vi "Measurement.vi"(0 "Position":T3(array[cluster]) {"Z" format="%.1f"; "Y" format="%.1f"; "X" format="%.1f"}, 1 "setup":T4=enum."Show Setup", 2 "Post Process":T2, 4 "File":T5, 5 "Results file":path, 7 "Raw data file":path, 11 "Setup filename":string) -> (14 "2nd plot":cluster{"X array":dbl[], "Y array":dbl[]}[](graph), 19 "Status Out":T1)   [LabVIEW 2013]
uses:
  Anemometry Sub Vis/Controls/Save_Data.ctl
  Anemometry Sub Vis/Controls/Setup.ctl
  Anemometry Sub Vis/Controls/Graph_Type.ctl
  Anemometry Sub Vis/Controls/Post_Process.ctl
  Anemometry Sub Vis/Gen Trav/Multi_Run_Status.ctl
  Anemometry Sub Vis/Controls/Inst_type.ctl
  ADAM Client/Sub VIs/ADAM Controls/Traverse_Level_State.ctl
  Anemometry Sub Vis/File/Setup_Filetype.ctl
  Anemometry Sub Vis/Globals/Trav_pos_global.vi
  Anemometry Sub Vis/Globals/Meas_global.vi
  Anemometry Sub Vis/Acquisition/PWA/PWAtasksGLOBAL.vi
  Anemometry Sub Vis/Acquisition/Data_Translation/DataTranslation_global.vi
  Anemometry Sub Vis/Globals/Preference_global.vi
  Anemometry Sub Vis/Globals/LDA_meas_global_1.vi
  Anemometry Sub Vis/Globals/LDA_meas_global_2.vi
  Anemometry Sub Vis/Globals/Dynamic_call_global.ph.vi
  Anemometry Sub Vis/Globals/Plug_in_data_global.vi
  Anemometry Sub Vis/Globals/Constants_global.vi
panel:
  out "Pause message":string
  out "Statistics":string[][](table)
  out "Actual Sampling freq":dbl=100.0 format="%.1f"
  in  "Desired Sampling freq (Hz)":dbl=100.0 format="%.1f"
  out "Current Block No":i32=5 caption="Current Block"
  in  "Pause":bool
  in  "No of Blocks":i32=5
  in  "stop":bool
  in  "No of samples":i32=1000 min=0 step=1
  in  "PP next block":bool
  in  "Tab Control":T6(tab)
  in  "Second Graph":T8={"Plot 1"=2, "Plot 2"=1, "Save graph"=0, "Plot Type"=enum."Vel histogram"} {"Save graph" items=["Do not save plot", "Save plot"]; "Plot 2" items=["Nothing", "U", "Volts", "Voltsr"]; "Plot 1" items=["Nothing", "U", "Volts", "Voltsr"]}
  in  "First Graph":T8={"Plot 1"=1, "Plot 2"=2, "Save graph"=0, "Plot Type"=enum."Velocity trace"} {"Save graph" items=["Do not save plot", "Save plot"]; "Plot 2" items=["Nothing", "U", "Volts", "Voltsr"]; "Plot 1" items=["Nothing", "U", "Volts", "Voltsr"]}
  out "First plot":cluster{"X array":dbl[], "Y array":dbl[]}[](graph)
  in  "Comments":string
  out "uv":dbl[][](graph)=[[-0.041806189081711534, -0.046435429052714985, -0.04035660097427599, -0.042187605126076694, -0.042052555599004206]]
  out "u^4":dbl[][](graph)
  out "u^3":dbl[][](graph)
  out "u^2":dbl[][](graph)=[[0.09743628875280319, 0.10575821456272283, 0.10126262927293661, 0.09890442087602569, 0.1022948212436432]]
  out "U":dbl[][](graph)=[[0.8295029456391334, 0.8915896983798417, 0.8415763502225625, 0.8394746126219594, 0.8466062785395404]]
  in  "Block average display control":cluster{"Name":string, "Include":bool}[](array[cluster])=[{"Name"="FF (C)", "Include"=FALSE}]
  in  "No of bins in histogram":i32=100
  out "Measurement time (min)":dbl=6.0 format="%.2f"
  in  "Correlate?":T9(ring)
  out "Diagnostic info":string[][](table)
  out "Array U":dbl[][](array[numeric]) format="%.2e"
  out "Array u^2":dbl[][](array[numeric]) format="%.2e"
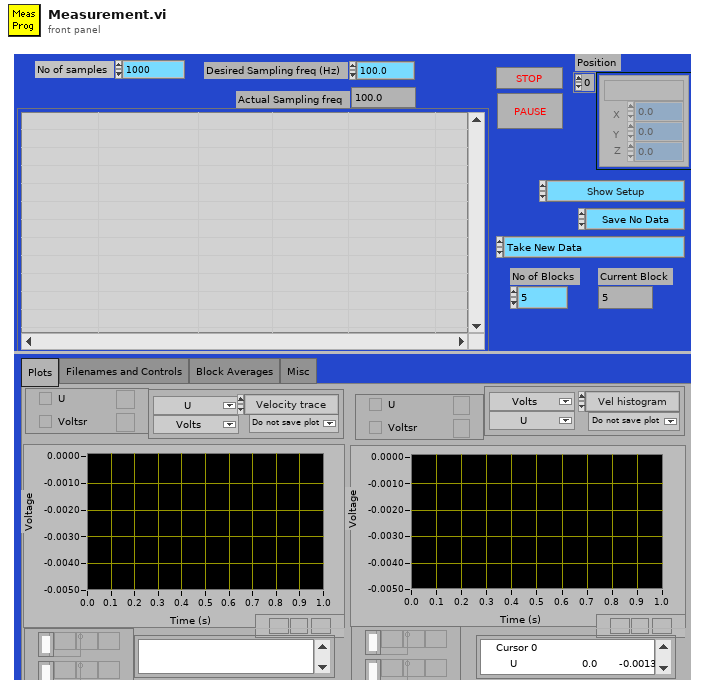
[diagram p1: front panel]
types:
  T1 = typedef "Multi_Run_Status.ctl" = enum16{"Continue", "Jump to Next Point", "Jump to Next Row", "Jump To Fall Back", "Terminate Run"}
  T2 = typedef "Post_Process.ctl" = enum16{"Take New Data", "Post Process Raw Data File"}
  T3 = cluster{"Name":string, "X":dbl, "Y":dbl, "Z":dbl}[]
  T4 = typedef "Setup.ctl" = enum16{"Run Program", "Show Setup", "Save Current Setup", "Setup Front Panel"}
  T5 = typedef "Save_Data.ctl" = enum16{"Save No Data", "Save Data"}
  T6 = enum32{"Plots", "Filenames and Controls", "Block Averages", "Misc"}
  T7 = typedef "Graph_Type.ctl" = enum16{"Show no graph", "Voltage trace", "Velocity trace", "Vel histogram", "Spectrum", "f.E(f) v Log f", "Auto-Corr"}
  T8 = cluster{"Plot 1":u16, "Plot 2":u16, "Save graph":u16, "Plot Type":T7}
  T9 = enum16{"Cross correlation off", "Show correlation panel", "Correlate without activating panel"}
  T10 = enum32{"Bad", "Idle", "Run top level", "Running"}
  T11 = cluster{"Name":string, "X":dbl, "Y":dbl, "Z":dbl}
  T12 = enum16{"Velocity", "Transit time", "Arrival time"}
  T13 = enum16{"Save no data", "Save data in new files", "Save data in existing files"}
  T14 = enum16{"Zero or one", "One", "Zero or more", "One or more"}
  T15 = cluster{"Weighting":dbl[], "Time (ms)":dbl[], "Voltage":dbl[], "Eng Values":dbl[]}
  T16 = typedef "Inst_type.ctl" = enum16{"Propeller anemometer", "Raw voltage", "Pressure Transducer", "Pitot-static tube", "Preston tube", "Hot wire", "Cross wire 1", "Cross wire 2", "Generic Linear", "Generic Polynomial", "Generic BackPoly", "Fast FID", "Thermocouple", "Cold wire", "Pulsed Wire", "LDA Vel", "LDA Tran time", "LDA Arr time"}
  T17 = typedef "Traverse_Level_State.ctl" = enum16{"Running", "Complete"}
  T18 = typedef "Setup_Filetype.ctl" = enum16{"Measurement Setups", "Calibration Setups", "General", "Results File Plotter Setups", "Speed Calib Tweaks"}
  T19 = typedef "Traverse_cluster.ctl" = cluster{"Start X":dbl, "Start Y":dbl, "Start Z":dbl, "End X":dbl, "End Y":dbl, "End Z":dbl, "No. of pts.":i32, "Spacing":T20, "Filename":path, "Tunnel Speed":dbl, "Averaging time (min)":dbl, "Extra Commands":string, "Specific Arguments":string, "Emission Rate (l/min)":dbl, "Trace Gas Concentration (%)":dbl, "Density Ratio":string, "Comments":string, "Row No":i32, "Row Type Selector":T21, "Completion time":string, "Row Duration (mins)":dbl, "No. of Valid pts.":i32, "Meas Setup File":string}
  T20 = typedef "Spacing.ctl" = enum16{"Linear", "Log", "Gauss", "Specified", "N/A"}
  T21 = typedef "Multi_run_mode.ctl" = enum16{"Move Traverse Only", "Set Tunnel Speed Only", "Set Source Only", "Set Measurement Conditions", "Single Measurement", "Vertical Profile", "Lateral Profile", "Longitudinal Profile", "Explore Volume", "Multi-Axis Profile", "Auto Calibrate", "Meas Fast FID Bkgnd", "Check Beam Power", "Scanning Valve Measurement", "Run VI Named:", "Set ADAM Ch", "Wait (minutes)", "Send Message", "Synchronize With:", "Fall Back to this Row", "Turn Off Row Repeating", "Blank Row", "Traverse 3D Volume"}
  T22 = typedef "Analysis_info_cluster.ctl" = cluster{"Colour":u32, "Inst type":T16, "Inst name":string, "Symbol":string, "Code name":string, "Extra Info":string, "Inst Array":T23, "Extra Titles":string[], "Extra Values":string[], "U":dbl, "u^2":dbl, "u^3":dbl, "u^4":dbl, "Skew_u":dbl, "Kurt_u":dbl, "Sd Error in Mean":dbl, "% u'/U":dbl, "X":dbl, "Y":dbl, "Z":dbl, "Timescale integral to 25%":dbl, "Sd Error in Variance":dbl, "Calib File":path, "Calib Constants":dbl[], "Output Position":bool, "Full Stats":bool, "Av Sampling Rate":dbl, "Av No of Samples":dbl, "Total Meas Time (s)":dbl, "ADAM Ch Name":string}
  T23 = typedef "Instrument_Array.ctl" = enum16{"PWA", "LDA", "Analogue"}
  T24 = typedef "LDA_Setup.ctl" = cluster{"dimensions":enum16{"1D", "2D"}, "Analogue Freq Multiplier":dbl}
  T25 = enum16{"Velocity", "Transit time", "Arrival time"}[]
  T26 = typedef "BSA_Type.ctl" = enum16{"57N11", "BSA F60"}
  T27 = typedef "BSA_info_Cluster.ctl" = cluster{"GPIB Address":string, "No of Check Bytes":i32, "Extra Info":string, "COLOUR":u32, "Wavelength (nm)":dbl}
  T28 = typedef "Ch_and_Spans.ctl" = cluster{"high limit (10V)":sgl, "low limit (-10V)":sgl, "Ch No":i16, "Var name":string, "Use Latest Calib":bool, "DAQmx Chan":tag}
  T29 = cluster{"Weighting":dbl[], "Time (ms)":dbl[], "Voltage":dbl[], "Eng Values":dbl[]}[]
  T30 = cluster{"Insts for plotting[0]":u16, "Insts for plotting[1]":u16}
  T31 = typedef "PWA_Data.ctl" = enum16{"No PWA Data", "One Ch PWA"}
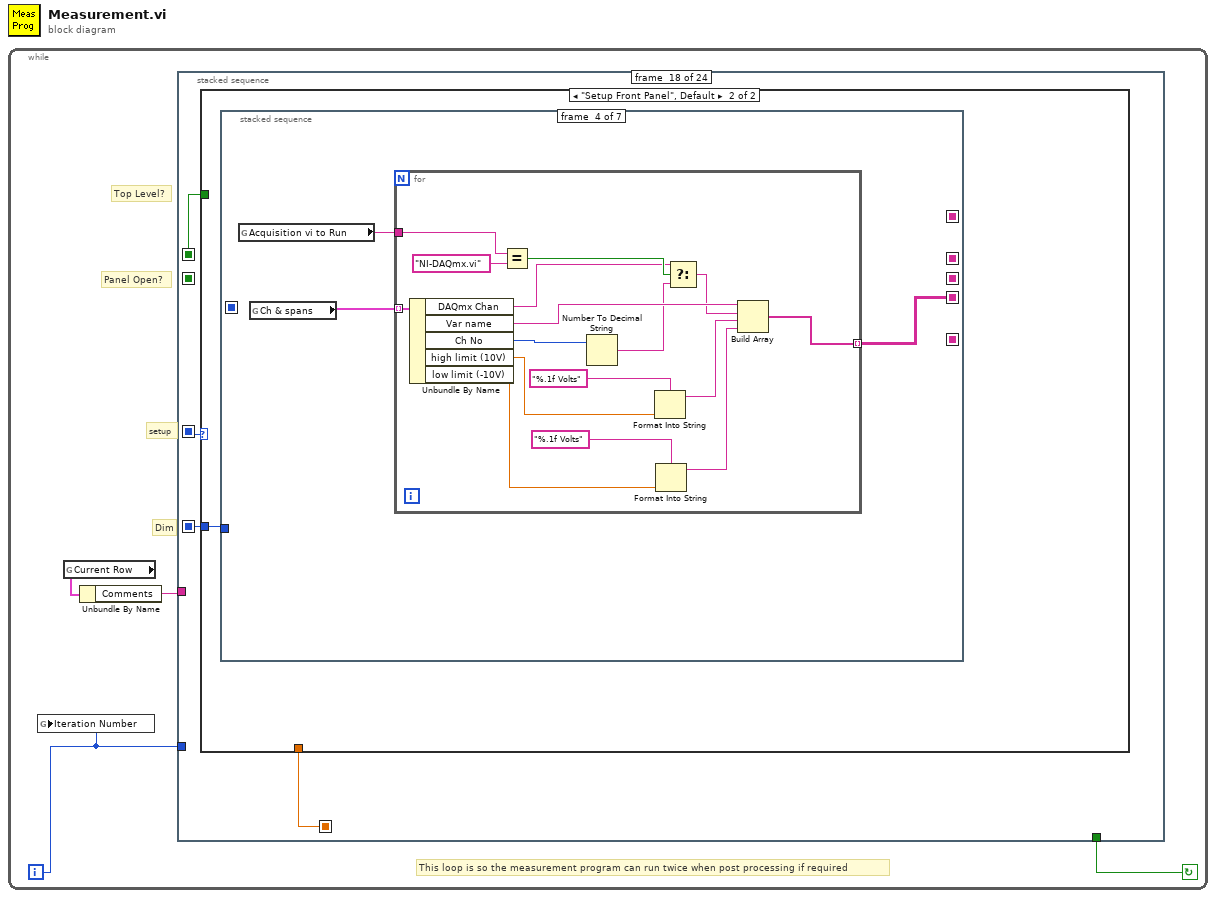
[diagram p0: block diagram]
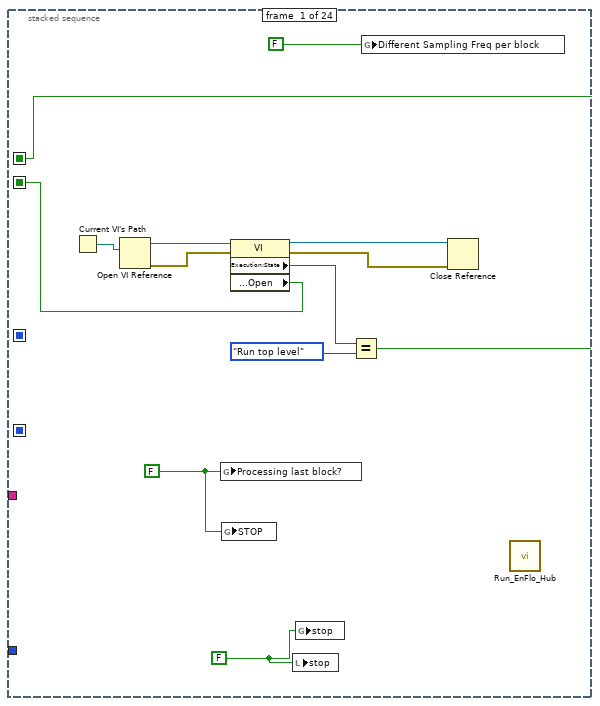
[diagram p2: hidden frame]
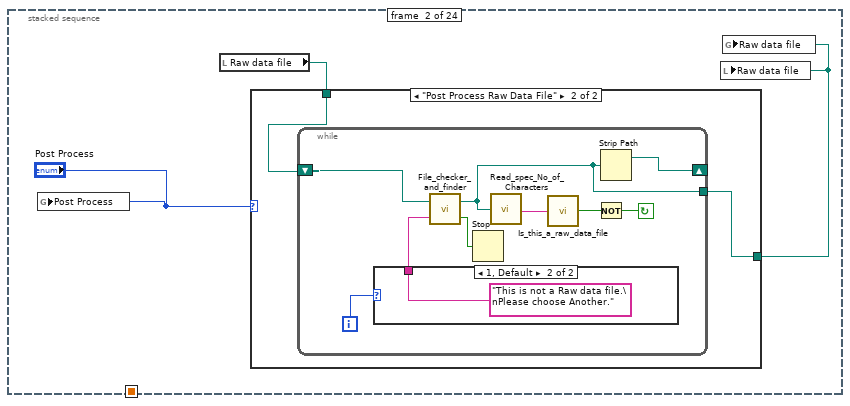
[diagram p3: hidden frame]
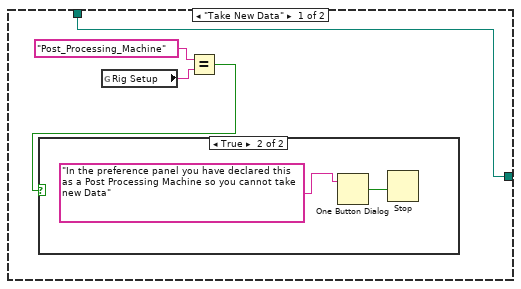
[diagram p4: hidden frame]
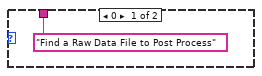
[diagram p6: hidden frame]
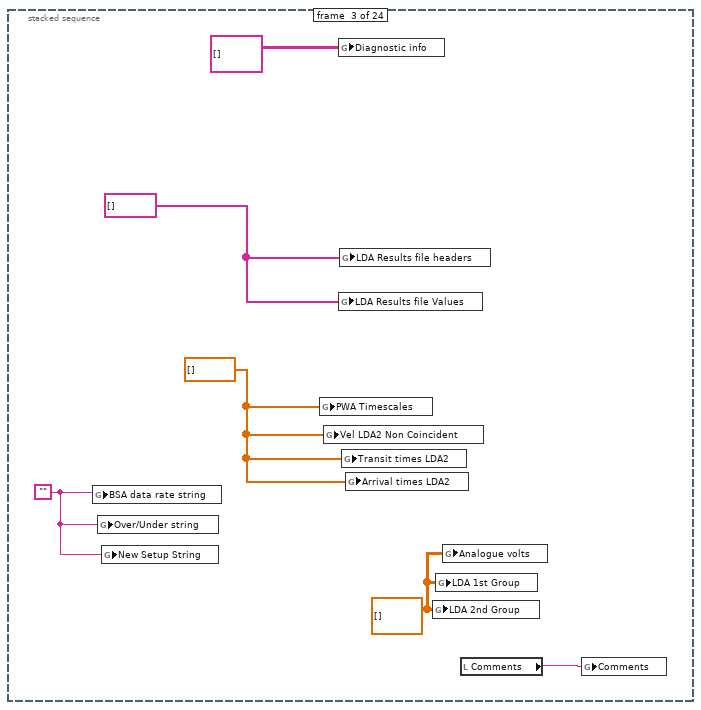
[diagram p7: hidden frame]
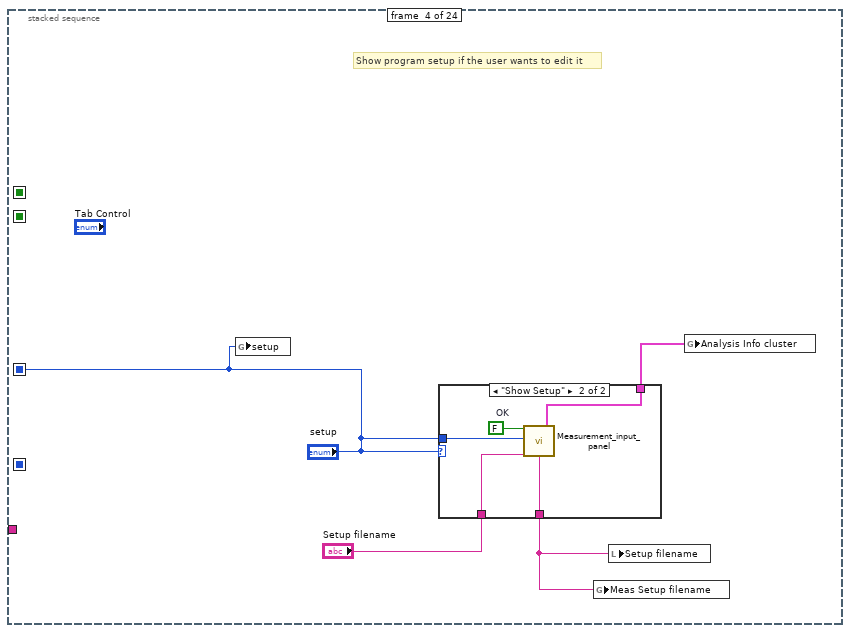
[diagram p8: hidden frame]
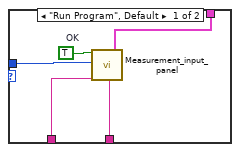
[diagram p9: hidden frame]
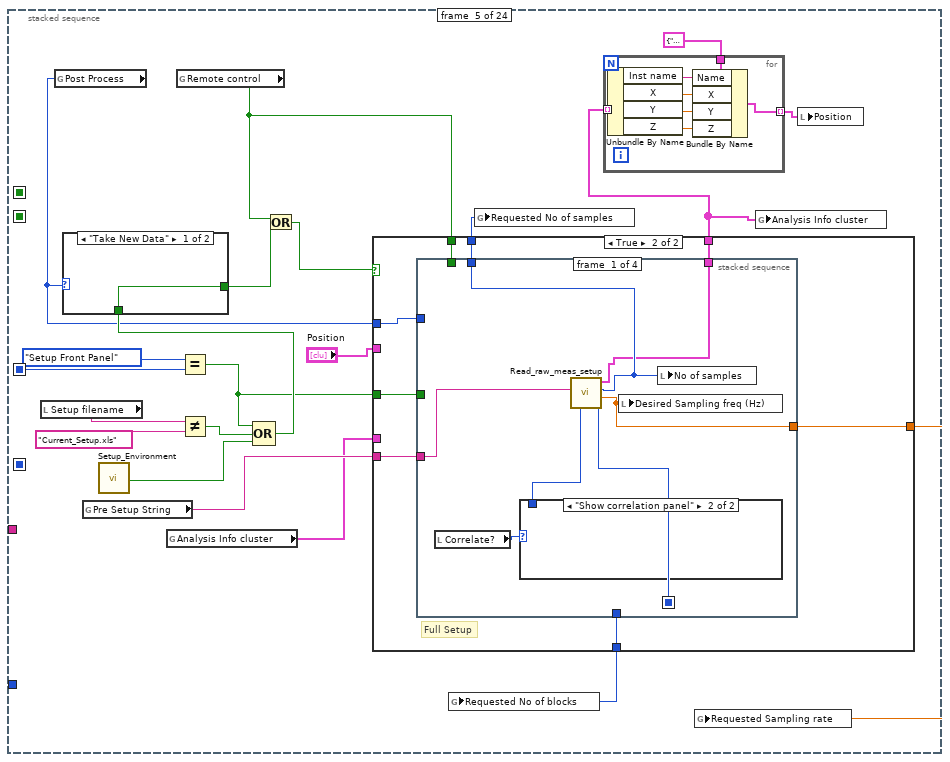
[diagram p10: hidden frame]
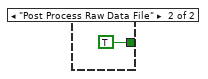
[diagram p11: hidden frame]
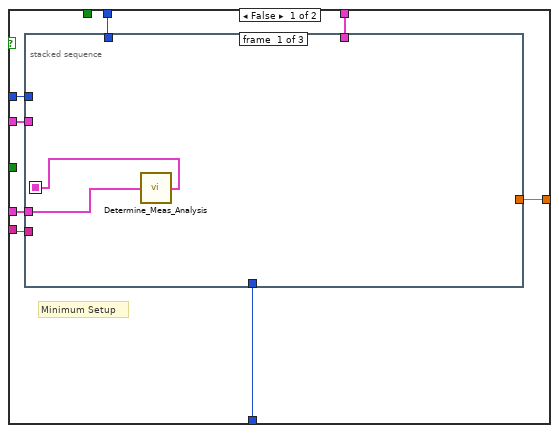
[diagram p12: hidden frame]
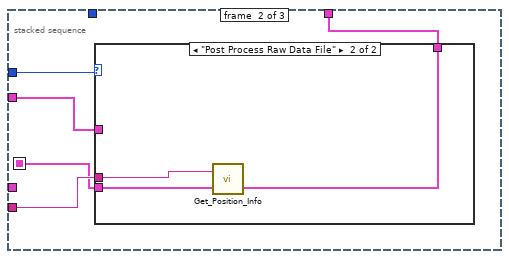
[diagram p13: hidden frame]
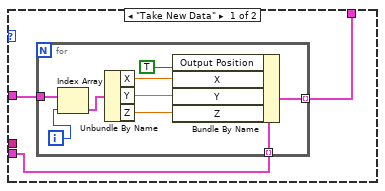
[diagram p14: hidden frame]
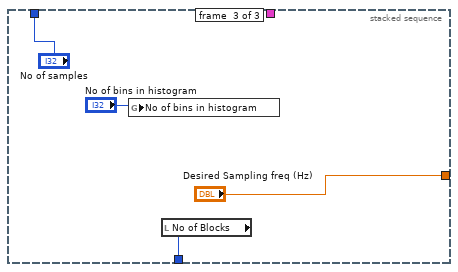
[diagram p15: hidden frame]
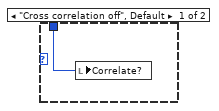
[diagram p16: hidden frame]
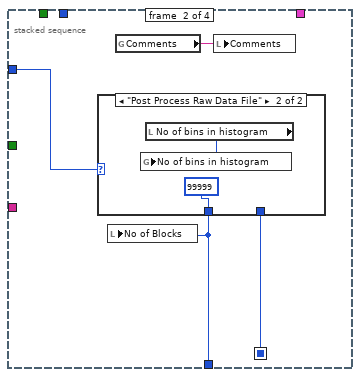
[diagram p17: hidden frame]
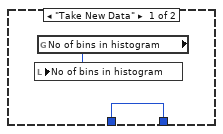
[diagram p18: hidden frame]
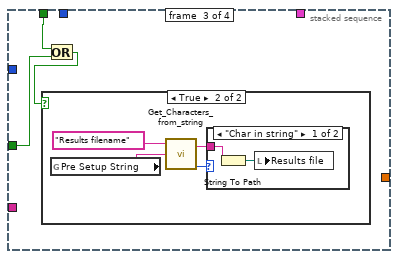
[diagram p19: hidden frame]
diagram:
  n1 = while {
    i -> [w1]
    stop <- w2 continue-if-true
    # "This loop is so the measurement program can run twice when post processing if required"
    # "Panel Open?"
    # "Top Level?"
    # "setup"
    # "Dim"
    n2 = global write "Meas_global.vi" "Iteration Number"(w1) -> ()
    n3 = global read "Trav_pos_global.vi" "Current Row"() -> (w3:T19)
    n4 = Unbundle By Name(w3) -> ("Comments"=w4:string)
    n5 = stacked-sequence {
      seq-local: [_ _ _ _ _ _ _ _ w202 _ _ _ _ _ _ _ _ _ _ _ _ _ _ _] -> [_ _ _ _ _ _ _ _ _ _ _ _ _ _ _ _ _ w752 _ _ _ _ _ _]
      seq-local: [_ _ _ "setup" _ _ _ _ _ _ _ _ _ _ _ _ _ _ _ _ _ _ _ _] -> [_ _ _ _ w71 _ _ _ w200 w289 _ _ _ _ w662 w682 w689 w753 w960 w1010 w1065 _ _ w1171]
      seq-local: [_ _ _ _ _ _ _ _ _ _ _ _ _ _ _ _ w685 _ _ _ _ _ _ _] -> [_ _ _ _ _ _ _ _ _ _ _ _ _ _ _ _ _ w751 w950 _ _ _ _ _]
      seq-local: [w7 _ _ _ _ _ _ _ _ _ _ _ _ _ _ _ _ _ _ _ _ _ _ _] -> [_ _ _ _ _ _ _ _ _ w269 _ _ _ _ w658 _ _ w750 _ _ _ _ _ _]
      seq-local: [w6 _ _ _ _ _ _ _ _ _ _ _ _ _ _ _ _ _ _ _ _ _ _ _] -> [_ _ _ _ _ _ _ _ _ _ _ _ w481 _ _ _ _ _ _ _ _ _ _ _]
      tunnel: w4 -> [_ _ _ _ _ _ _ w197 _ _ _ _ _ _ _ _ _ _ _ _ _ _ w1140 _]
      tunnel: w1 -> [_ _ _ _ _ _ _ _ _ _ _ _ _ _ _ _ _ _ _ _ _ _ w1135 _]
      tunnel: [_ _ _ _ _ _ _ _ _ _ _ _ _ _ _ _ _ _ _ _ _ _ w1134 _] -> w2
      frame #0 {
        w15 = FALSE ("Processing last block?")
        w16 = FALSE ("stop")
        n6 = Current VI's Path() -> (path=w8:path)
        n7 = Open VI Reference(vi path=w8) -> (vi reference=w9:refnum<vi>, error out=w10:errorcluster)  [unwired: 1 in, 4 out]
        n8 = global write "Meas_global.vi" "Processing last block?"(w15) -> ()
        n9 = global write "PWAtasksGLOBAL.vi" "STOP"(w15) -> ()
        n10 = property class="VI"(reference=w9, error in=w10) -> (reference out=w11:refnum<vi>, error out=w12:errorcluster, "Execution:State"=w13:T10, "Front Panel.Open"=w6:bool)
        n11 = local write "stop"(w16) -> ()
        n12 = global write "Meas_global.vi" "stop"(w16) -> ()
        n13 = Equal?(x=w13, y=T10."Run top level" ("Exec.State")) -> (x = y?=w7:bool)
        n14 = global write "DataTranslation_global.vi" "Different Sampling Freq per block"(FALSE ("Different Sampling Freq per block")) -> ()
        n15 = Close Reference(reference=w11, error in (no error)=w12) -> ()  [unwired: 1 out]
        n16 = call "Run_EnFlo_Hub.vi"() -> ()  [unwired: 8 out]
      }
      frame #1 {
        n17 = global write "Meas_global.vi" "Post Process"("Post Process") -> ()
        n18 = local read "Raw data file"() -> (w19:path)
        n19 = case shown="\"Post Process Raw Data File\"" "Post Process" {
          tunnel: [w23 w27] -> w18
          tunnel: w19 -> [w23 w26]
          frame "Take New Data" {
            n20 = global read "Preference_global.vi" "Rig Setup"() -> (w22:string)
            n21 = Equal?(x="Post_Processing_Machine" ("Rig Setup"), y=w22) -> (x = y?=w20:bool)
            n22 = case shown="True" w20 {
              frame False {
              }
              frame True {
                n23 = One Button Dialog(message="In the preference panel you have declared this as a Post Processing Machine so you cannot take new Data") -> (true=w24:bool)  [unwired: 1 in]
                n24 = Stop(stop? (T)=w24) -> ()
              }
            }
          }
          frame "Post Process Raw Data File" {
            n25 = while {
              tunnel: [w29] -> w27
              shift-left: w26 -> [w31]
              shift-right: [w30] -> _
              i -> [w32]
              stop <- w33 continue-if-true
              n26 = case shown="1, Default" w32 {
                tunnel: ["Find a Raw Data File to Post Process" ("Promp if not found") "This is not a Raw data file.\nPlease choose Another." ("Promp if not found")] -> w36
                frame 0 {
                }
                frame 1, Default {
                }
              }
              n27 = call "File_checker_and_finder.vi"("Promp if not found"=w36, "Filename In"=w31) -> ("cancelled"=w28:bool, "Filename Out"=w29:path)
              n28 = Stop(stop? (T)=w28) -> ()
              n29 = call "Read_spec_No_of_Characters.vi"("Filename"=w29) -> ("character string"=w35:string)  [unwired: 1 out]
              n30 = call "Is_this_a_raw_data_file.vi"("character string"=w35) -> ("Raw Dat File?"=w34:bool)  [unwired: 2 out]
              n31 = Not(x=w34) -> (.not. x?=w33:bool)
              n32 = Strip Path(path=w29) -> (stripped path=w30:path)  [unwired: 1 out]
            }
          }
        }
        n33 = local write "Raw data file"(w18) -> ()
        n34 = global write "Meas_global.vi" "Raw data file"(w18) -> ()
      }
      frame #2 {
        w39 = dbl[][] [] ("LDA 2nd Group")
        w40 = dbl[] [] ("LDA Timescales")
        w42 = string[] [] ("Plug in values")
        w44 = ""
        n35 = global write "Meas_global.vi" "BSA data rate string"(w44) -> ()
        n36 = global write "Meas_global.vi" "Over/Under string"(w44) -> ()
        n37 = global write "Meas_global.vi" "New Setup String"(w44) -> ()
        n38 = global write "PWAtasksGLOBAL.vi" "PWA Timescales"(w40) -> ()
        n39 = global write "LDA_meas_global_2.vi" "Vel LDA2 Non Coincident"(w40) -> ()
        n40 = global write "Meas_global.vi" "Diagnostic info"(string[][] [] ("Diagnostic info")) -> ()
        n41 = global write "LDA_meas_global_1.vi" "LDA Results file Values"(w42) -> ()
        n42 = global write "LDA_meas_global_1.vi" "LDA Results file headers"(w42) -> ()
        n43 = global write "LDA_meas_global_2.vi" "Transit times LDA2"(w40) -> ()
        n44 = global write "LDA_meas_global_2.vi" "Arrival times LDA2"(w40) -> ()
        n45 = global write "LDA_meas_global_2.vi" "LDA 2nd Group"(w39) -> ()
        n46 = global write "LDA_meas_global_2.vi" "LDA 1st Group"(w39) -> ()
        n47 = global write "Meas_global.vi" "Analogue volts"(w39) -> ()
        n48 = local read "Comments"() -> (w43:string)
        n49 = global write "Meas_global.vi" "Comments"(w43) -> ()
      }
      frame #3 {
        # "Show program setup if the user wants to edit it"
        n50 = global write "Meas_global.vi" "setup"("setup") -> ()
        n51 = case shown="\"Show Setup\"" "setup" {
          tunnel: [w52 w57] -> w48
          tunnel: "Setup filename" -> [w51 w56]
          tunnel: [w50 w55] -> w46
          tunnel: "setup" -> [w49 w54]
          frame "Run Program", Default {
            w53 = TRUE  # OK
            n52 = call "Measurement_input_panel.vi"("OK"=w53, "setup"=w49, "Setup filename"=w51) -> ("Setup filename out"=w50:string, "Analysis Info cluster"=w52:T22[])  [unwired: 15 out]
          }
          frame "Show Setup" {
            w58 = FALSE  # OK
            n53 = call "Measurement_input_panel.vi"("OK"=w58, "setup"=w54, "Setup filename"=w56) -> ("Setup filename out"=w55:string, "Analysis Info cluster"=w57:T22[])  [unwired: 15 out]
          }
        }
        n54 = global write "Meas_global.vi" "Meas Setup filename"(w46) -> ()
        n55 = local write "Setup filename"(w46) -> ()
        n56 = global write "Meas_global.vi" "Analysis Info cluster"(w48) -> ()
      }
      frame #4 {
        n57 = local read "Setup filename"() -> (w75:string)
        n58 = global read "Meas_global.vi" "Post Process"() -> (w70:T2)
        n59 = global read "Meas_global.vi" "Pre Setup String"() -> (w66:string)
        n60 = call "Setup_Environment.vi"() -> ("First Time"=w67:bool)  [unwired: 1 in]
        n61 = global read "Meas_global.vi" "Analysis Info cluster"() -> (w63:T22[])
        n62 = global read "Meas_global.vi" "Remote control"() -> (w65:bool)
        n63 = Equal?(x=Setup."Setup Front Panel" ("setup"), y=w71) -> (x = y?=w64:bool)
        n64 = Not Equal?(x=w75, y="Current_Setup.xls" ("Setup filename")) -> (x != y?=w73:bool)
        n65 = Compound Arithmetic op=OR(w64, w73, w67) -> (w72:bool)
        n66 = case shown="\"Take New Data\"" w70 {
          tunnel: [w87 TRUE] -> w79
          tunnel: w72 -> [w87 _]
          frame "Take New Data" {
          }
          frame "Post Process Raw Data File" {
          }
        }
        n67 = Or(x=w65, y=w79) -> (x .or. y?=w78:bool)
        n68 = case shown="True" w78 {
          tunnel: w70 -> [w92 w130]
          tunnel: [w96 w129] -> w68
          tunnel: [w95 w124] -> w77
          tunnel: [w94 w128] -> w76
          tunnel: [w93 w127] -> w62
          tunnel: w66 -> [w91 w126]
          tunnel: "Position" -> [w90 _]
          tunnel: w65 -> [_ w125]
          tunnel: w64 -> [_ w123]
          tunnel: w63 -> [w89 _]
          frame False {
            # "Minimum Setup"
            n69 = stacked-sequence {
              seq-local: [w97 _ _] -> [_ w99 _]
              tunnel: [_ _ "Desired Sampling freq (Hz)"] -> w96
              tunnel: [_ _ w121] -> w95
              tunnel: [_ _ "No of samples"] -> w94
              tunnel: [_ w102 _] -> w93
              tunnel: w92 -> [_ w103 _]
              tunnel: w91 -> [_ w101 _]
              tunnel: w90 -> [_ w100 _]
              tunnel: w89 -> [w98 _ _]
              frame #0 {
                n70 = call "Determine_Meas_Analysis.vi"("Analysis info Cluster In"=w98) -> ("Analysis info Cluster Out"=w97:T22[])
              }
              frame #1 {
                n71 = case shown="\"Post Process Raw Data File\"" w103 {
                  tunnel: [w104 w116] -> w102
                  tunnel: w100 -> [w106 _]
                  tunnel: w101 -> [_ w117]
                  tunnel: w99 -> [w105 w118]
                  frame "Take New Data" {
                    n72 = for {
                      tunnel: w106 -> [w109]
                      tunnel: w105 -> [w115] mode=indexing
                      tunnel: [w111] -> w104 mode=indexing
                      i -> [w110]
                      n73 = Index Array(array=w109, index=w110) -> (element=w108:T11)
                      n74 = Unbundle By Name(w108) -> ("X"=w112:dbl, "Y"=w113:dbl, "Z"=w114:dbl)
                      n75 = Bundle By Name(cluster=w115, "Output Position"=TRUE, "X"=w112, "Y"=w113, "Z"=w114) -> (w111:T22)
                    }
                  }
                  frame "Post Process Raw Data File" {
                    n76 = call "Get_Position_Info.vi"("Analysis Info cluster"=w118, "Setup file string"=w117) -> ("Analysis Info cluster 2"=w116:T22[])  [unwired: 1 in]
                  }
                }
              }
              frame #2 {
                n77 = global write "Meas_global.vi" "No of bins in histogram"("No of bins in histogram") -> ()
                n78 = local read "No of Blocks"() -> (w121:i32)
              }
            }
          }
          frame True {
            # "Full Setup"
            n79 = stacked-sequence {
              seq-local: [w134 _ _ _] -> [_ w140 _ _]
              tunnel: w130 -> [_ w141 _ w156]
              tunnel: [w137 _ _ _] -> w129
              tunnel: [w136 _ _ _] -> w128
              tunnel: [w133 _ _ _] -> w127
              tunnel: w126 -> [w135 _ _ _]
              tunnel: w125 -> [_ _ w149 _]
              tunnel: [_ w139 _ _] -> w124
              tunnel: w123 -> [_ _ w148 _]
              frame #0 {
                n80 = local read "Correlate?"() -> (w132:T9)
                n81 = call "Read_raw_meas_setup.vi"("Setup file string"=w135) -> ("No of Blocks"=w134:i32, "Sampling freq (Hz)"=w137:dbl, "No of samples"=w136:i32, "Analysis Info cluster 2"=w133:T22[], "Correlate?"=w131:T9)  [unwired: 4 out]
                n82 = case shown="\"Show correlation panel\"" w132 {
                  tunnel: w131 -> [w138 _]
                  frame "Cross correlation off", Default {
                    n83 = local write "Correlate?"(w138) -> ()
                  }
                  frame "Show correlation panel" {
                  }
                }
                n84 = local write "Desired Sampling freq (Hz)"(w137) -> ()
                n85 = local write "No of samples"(w136) -> ()
              }
              frame #1 {
                n86 = case shown="\"Post Process Raw Data File\"" w141 {
                  tunnel: [w144 99999 ("No of Blocks")] -> w139
                  tunnel: w140 -> [w144 _]
                  frame "Take New Data" {
                    n87 = global read "Meas_global.vi" "No of bins in histogram"() -> (w143:i32)
                    n88 = local write "No of bins in histogram"(w143) -> ()
                  }
                  frame "Post Process Raw Data File" {
                    n89 = local read "No of bins in histogram"() -> (w145:i32)
                    n90 = global write "Meas_global.vi" "No of bins in histogram"(w145) -> ()
                  }
                }
                n91 = local write "No of Blocks"(w139) -> ()
                n92 = global read "Meas_global.vi" "Comments"() -> (w142:string)
                n93 = local write "Comments"(w142) -> ()
              }
              frame #2 {
                n94 = Or(x=w149, y=w148) -> (x .or. y?=w147:bool)
                n95 = case shown="True" w147 {
                  frame False {
                  }
                  frame True {
                    n96 = global read "Meas_global.vi" "Pre Setup String"() -> (w150:string)
                    n97 = call "Get_Characters_from_string.vi"("Input string"=w150, "Variable name"="Results filename") -> ("Status"=w153:enum16{"Char in string", "Char not in string"}, "Value"=w152:string)  [unwired: 1 in]
                    n98 = case shown="\"Char in string\"" w153 {
                      tunnel: w152 -> [w155 _]
                      frame "Char in string" {
                        n99 = String To Path(string=w155) -> (path=w154:path)
                        n100 = local write "Results file"(w154) -> ()
                      }
                      frame "Char not in string" {
                      }
                    }
                  }
                }
              }
              frame #3 {
                n101 = case shown="\"Take New Data\"" w156 {
                  frame "Take New Data" {
                    n102 = global read "Meas_global.vi" "Second Graph"() -> (w157:T8)
                    n103 = global read "Meas_global.vi" "First Graph"() -> (w158:T8)
                    n104 = local write "Second Graph"(w157) -> ()
                    n105 = local write "First Graph"(w158) -> ()
                  }
                  frame "Post Process Raw Data File" {
                  }
                }
              }
            }
          }
        }
        n106 = global write "Meas_global.vi" "Requested No of blocks"(w77) -> ()
        n107 = global write "Meas_global.vi" "Requested No of samples"(w76) -> ()
        n108 = for {
          tunnel: w62 -> [w86] mode=indexing
          tunnel: [w82] -> w60 mode=indexing
          tunnel: T11 {"Name"="", "X"=0.0, "Y"=0.0, "Z"=0.0} ("Position") -> [w81]
          n109 = Unbundle By Name(w86) -> ("Inst name"=w80:string, "X"=w83:dbl, "Y"=w84:dbl, "Z"=w85:dbl)
          n110 = Bundle By Name(cluster=w81, "Name"=w80, "X"=w83, "Y"=w84, "Z"=w85) -> (w82:T11)
        }
        n111 = global write "Meas_global.vi" "Requested Sampling rate"(w68) -> ()
        n112 = global write "Meas_global.vi" "Analysis Info cluster"(w62) -> ()
        n113 = local write "Position"(w60) -> ()
      }
      frame #5 {
        n114 = global read "Meas_global.vi" "Post Process"() -> (w159:T2)
        n115 = case shown="\"Post Process Raw Data File\"" w159 {
          tunnel: [w162 w163] -> w160
          frame "Take New Data" {
            n116 = Get Date/Time In Seconds() -> (seconds since 1Jan1904=w161:timestamp)
            n117 = To Double Precision Float(number=w161) -> (double precision float=w162:dbl)
          }
          frame "Post Process Raw Data File" {
            n118 = global read "Meas_global.vi" "Pre Setup String"() -> (w166:string)
            n119 = call "Get_Characters_from_string.vi"("Input string"=w166, "Variable name"="Seconds since 1/1/04") -> ("Value"=w164:string)  [unwired: 1 in, 1 out]
            n120 = call "String_2_Number.vi"("Value"=w164) -> ("Numeric"=w163:dbl)
          }
        }
        n121 = global write "Meas_global.vi" "Time Data was Aquired"(w160) -> ()
      }
      frame #6 {
        n122 = global read "Dynamic_call_global.ph.vi" "Initial Plug Ins"() -> (w168:string[])
        n123 = global read "Dynamic_call_global.ph.vi" "Initial Plug Ins Extra"() -> (w169:string[])
        n124 = Build Array (concatenate)(w169, w168) -> (w167:string[])
        n125 = Array Size(array=w167) -> (size(s)=w171:i32)
        n126 = Greater Than 0?(x=w171) -> (x > 0?=w170:bool)
        n127 = case shown="True" w170 {
          tunnel: w167 -> [_ w172]
          frame False {
          }
          frame True {
            n128 = stacked-sequence {
              tunnel: w172 -> [w174 _]
              frame #0 {
                n129 = global read "Meas_global.vi" "Post Process"() -> (w176:T2)
                n130 = call "Plug_in_Directories.vi"() -> ("Initial"=w173:path)  [unwired: 3 out]
                n131 = Equal?(x=w176, y=Post_Process."Post Process Raw Data File" ("Post Process")) -> (x = y?=w175:bool)
                n132 = for {
                  tunnel: w175 -> [w182]
                  tunnel: w174 -> [w179] mode=indexing
                  tunnel: w173 -> [w178]
                  w189 = FALSE  # Dialog Box (T)
                  n133 = Build Path(base path=w178, name or relative path=w179) -> (appended path=w180:path)
                  n134 = Open VI Reference(vi path=w180) -> (vi reference=w187:refnum<vi>, error out=w186:errorcluster)  [unwired: 2 in, 3 out]
                  n135 = property class="VI"(reference=w187, error in=w186, "Front Panel Window:Open"=TRUE ("Wait until done")) -> (reference out=w185:refnum<vi>, error out=w184:errorcluster)
                  n136 = invoke class="VI" method="Run VI"(reference=w185, error in=w184, "Wait until done"=w182, "Auto Dispose Ref"=FALSE) -> (reference out=w192:refnum<vi>, error out=w191:errorcluster)  [unwired: 1 in, 3 out]
                  n137 = Close Reference(reference=w192, error in (no error)=w191) -> (error out=w190:errorcluster)
                  n138 = call "EnFlo_Error_Handler.vi"("error in (no error)"=w190, "Error Type"="Launching Initial Plug In", "Dialog Box (T)"=w189) -> ()  [unwired: 3 out]
                }
              }
              frame #1 {
                n139 = global read "Meas_global.vi" "Requested No of blocks"() -> (w194:i32)
                n140 = global read "Meas_global.vi" "Comments"() -> (w193:string)
                n141 = local write "Comments"(w193) -> ()
                n142 = local write "No of Blocks"(w194) -> ()
              }
            }
          }
        }
      }
      frame #7 {
        n143 = local read "Comments"() -> (w198:string)
        n144 = Concatenate Strings(w197, w198) -> (w196:string)
        n145 = call "Text_without_format.vi"("Input string"=w196) -> ("Output string"=w195:string)
        n146 = local write "Comments"(w195) -> ()
        n147 = global write "Meas_global.vi" "Comments"(w195) -> ()
      }
      frame #8 {
        n148 = global read "Meas_global.vi" "LDA set up"() -> (w203:T24)
        n149 = Unbundle By Name(w203) -> ("dimensions"=w202:enum16{"1D", "2D"})
        n150 = global read "Meas_global.vi" "LDA data"() -> (w210:enum16{"No LDA data", "Take LDA data"})
        n151 = global read "Meas_global.vi" "Post Process"() -> (w212:T2)
        n152 = Not Equal?(x=w200, y=Setup."Setup Front Panel" ("setup")) -> (x != y?=w199:bool)
        n153 = Equal?(x=w200, y=Setup."Show Setup" ("setup")) -> (x = y?=w204:bool)
        n154 = Equal?(x=w210, y=enum16{"No LDA data", "Take LDA data"}."Take LDA data" ("LDA data")) -> (x = y?=w206:bool)
        n155 = Equal?(x=w212, y=Post_Process."Take New Data" ("Post Process")) -> (x = y?=w207:bool)
        n156 = Compound Arithmetic op=AND(w199, w206, w207) -> (w205:bool)
        n157 = case shown="True" w205 {
          tunnel: w202 -> [_ w221]
          tunnel: w200 -> [_ w220]
          tunnel: w204 -> [_ w218]
          frame False {
            n158 = Build Array(T12."Velocity", T12."Transit time", T12."Arrival time") -> (w213:T25)
            n159 = global write "LDA_meas_global_1.vi" "Number of measured quantities"(3 ("Number of measured quantities")) -> ()
            n160 = global write "LDA_meas_global_2.vi" "data type"(w213) -> ()
            n161 = global write "LDA_meas_global_1.vi" "data type"(w213) -> ()
          }
          frame True {
            n162 = global read "LDA_meas_global_1.vi" "BSA Type"() -> (w219:T26)
            n163 = case shown="\"57N11\"" w219 {
              tunnel: w221 -> [w223 _]
              tunnel: w220 -> [w222 _]
              tunnel: w218 -> [_ w259]
              frame "57N11" {
                n164 = stacked-sequence {
                  tunnel: w223 -> [w226 w252]
                  tunnel: w222 -> [w225 _]
                  frame #0 {
                    n165 = global read "Meas_global.vi" "Remote control"() -> (w224:bool)
                    n166 = case shown="\"2D\"" w226 {
                      tunnel: w225 -> [w228 w241]
                      tunnel: w224 -> [w227 w240]
                      frame "2D" {
                        n167 = while {
                          tunnel: w227 -> [w229]
                          tunnel: w228 -> [w230]
                          stop <- w231 continue-if-true
                          n168 = stacked-sequence {
                            tunnel: [_ _ w237] -> w231
                            tunnel: w230 -> [w232 w234 _]
                            tunnel: w229 -> [_ _ w236]
                            frame #0 {
                              w233 = "1"  # BSA Number
                              n169 = call "Control_BSA_setup.vi"("setup"=w232, "BSA number"=w233) -> ()  [unwired: 14 out]
                            }
                            frame #1 {
                              w235 = "2"  # BSA Number
                              n170 = call "Control_BSA_setup.vi"("setup"=w234, "BSA number"=w235) -> ()  [unwired: 14 out]
                            }
                            frame #2 {
                              n171 = case shown="False" w236 {
                                tunnel: [w238 FALSE ("ok")] -> w237
                                frame False {
                                n172 = call "BSA_setup_check.vi"() -> ("ok"=w238:bool)
                                }
                                frame True {
                                }
                              }
                            }
                          }
                        }
                      }
                      frame "1D" {
                        n173 = stacked-sequence {
                          tunnel: w241 -> [w242 _]
                          tunnel: w240 -> [_ _]
                          frame #0 {
                            w243 = "1"  # BSA Number
                            n174 = call "Control_BSA_setup.vi"("setup"=w242, "BSA number"=w243) -> ()  [unwired: 14 out]
                          }
                          frame #1 {
                            n175 = global read "LDA_meas_global_2.vi" "BSA2 info"() -> (w244:T27)
                            n176 = Unbundle By Name(w244) -> ("GPIB Address"=w245:string)
                            n177 = call "Set_BSA_Coincidence.vi"("GPIB address"=w245, "Set Coincidence"=enum16{"Slave", "Master", "Private"}."Slave") -> ()  [unwired: 1 in, 5 out]
                          }
                        }
                      }
                    }
                  }
                  frame #1 {
                    n178 = global read "Meas_global.vi" "Remote control"() -> (w250:bool)
                    n179 = Equal?(x=w252, y=enum16{"1D", "2D"}."2D" ("dimensions")) -> (x = y?=w248:bool)
                    n180 = Not(x=w250) -> (.not. x?=w249:bool)
                    n181 = And(x=w249, y=w248) -> (x .and. y?=w247:bool)
                    n182 = case shown="True" w247 {
                      frame False {
                      }
                      frame True {
                        n183 = global read "LDA_meas_global_1.vi" "BSA1 info"() -> (w254:T27)
                        n184 = global read "LDA_meas_global_2.vi" "BSA2 info"() -> (w255:T27)
                        n185 = Build Array(w254, w255) -> (w253:T27[])
                        n186 = for {
                          tunnel: w253 -> [w257] mode=indexing
                          n187 = Unbundle By Name(w257) -> ("GPIB Address"=w256:string)
                          n188 = call "Set_BSA_Coincidence.vi"("GPIB address"=w256, "Set Coincidence"=enum16{"Slave", "Master", "Private"}."Master") -> ()  [unwired: 1 in, 5 out]
                        }
                      }
                    }
                  }
                }
              }
              frame "BSA F60" {
                n189 = disable-structure shown="TARGET_TYPE==Windows" {
                  disable-tunnel: w259 -> [_ w260]
                  frame condition #0 {
                  }
                  frame condition #1 (active) {
                    n190 = while {
                      tunnel: w260 -> [w263]
                      stop <- w261 continue-if-true
                      n191 = call "Edit_BSA_IP.vi"("Show Panel"=w263) -> ("Run LDA Diagnostic Out"=w262:bool)  [unwired: 2 out]
                      n192 = case shown="True" w262 {
                        tunnel: [FALSE w265] -> w261
                        frame False {
                        }
                        frame True {
                          n193 = call "F60_Diagnostic.vi"() -> ("Edit BSA Setup Out"=w265:bool)  [unwired: 11 in]
                        }
                      }
                    }
                  }
                }
              }
            }
          }
        }
      }
      frame #9 {
        w274 = Save_Data."Save No Data" ("File")
        w290 = Post_Process."Take New Data"  # Post Process
        n194 = global read "Trav_pos_global.vi" "Meas Setup Number"() -> (w270:i32)
        n195 = Not Equal?(x=Setup."Run Program" ("setup"), y=w289) -> (x != y?=w275:bool)
        n196 = call "Current_Filepath.vi"("Filename in"="Results file", "Data Type"="Results") -> ("Filename Out"=w268:path)  [unwired: 1 out]
        n197 = global read "Meas_global.vi" "Remote control"() -> (w286:bool)
        n198 = global read "Meas_global.vi" "Post Process"() -> (w277:T2)
        n199 = Equal?(x="File", y=w274) -> (x = y?=w284:bool)
        n200 = case shown="1, Default" w270 {
          tunnel: [w293 w295] -> w271
          tunnel: w268 -> [w293 w302]
          tunnel: w270 -> [_ w303]
          frame 0 {
          }
          frame 1, Default {
            n201 = Add(x=96, y=w303) -> (x+y=w305:i32)
            n202 = Build Array(w305) -> (w306:i32[])
            n203 = Strip Path(path=w302) -> (stripped path=w296:path, name=w301:string)
            n204 = Byte Array To String(unsigned byte array=w306) -> (string=w299:string)
            n205 = call "Add_filename_suffix.vi"("Filename"=w301) -> ("Original Suffix"=w298:string, "Base name"=w300:string)  [unwired: 1 in, 2 out]
            n206 = Format Into String(format string="%s_%s%s", w300, w299, w298) -> (resulting string=w297:string)  [unwired: 2 in, 1 out]
            n207 = Build Path(base path=w296, name or relative path=w297) -> (appended path=w295:path)
          }
        }
        n208 = Equal?(x=w277, y=w290) -> (x = y?=w276:bool)
        n209 = And(x=w286, y=w276) -> (x .and. y?=w282:bool)
        n210 = Compound Arithmetic op=AND(w284, invert w286, w276, invert w275) -> (w285:bool)
        n211 = while {
          shift-left: _ -> [w311]
          shift-right: [w308] -> _
          tunnel: "File" -> [w309]
          tunnel: [w312] -> w283
          tunnel: w285 -> [w308]
          stop <- FALSE continue-if-true
          n212 = Compound Arithmetic op=AND(w308, invert w311) -> (w310:bool)
          n213 = case shown="True" w310 {
            tunnel: [w313 w316] -> w312
            tunnel: w309 -> [w313 _]
            frame False {
            }
            frame True {
              n214 = Two Button Dialog(message="Do you wish to save the data?", 1:"Save Data" ("F button name (\"Cancel\")"), 2:"Save No Data" ("T button name (\"OK\")")) -> (T button?=w317:bool)
              n215 = Select(t=Save_Data."Save No Data" ("File"), s=w317, f=Save_Data."Save Data" ("File")) -> (s? t:f=w316:T5)
            }
          }
        }
        n216 = Equal?(x=w274, y=w283) -> (x = y?=w273:bool)
        n217 = Or(x=w273, y=w275) -> (x .or. y?=w288:bool)
        n218 = case shown="False" w288 {
          tunnel: w271 -> [w332 w340]
          tunnel: [w331 w340] -> w291
          tunnel: "Raw data file" -> [w330 w341]
          tunnel: [w325 w341] -> w280
          tunnel: w289 -> [w329 _]
          tunnel: w283 -> [w328 _]
          tunnel: [w326 T13."Save no data" ("File output")] -> w278
          tunnel: [w327 w338] -> w272
          tunnel: w282 -> [_ w335]
          tunnel: w275 -> [_ w334]
          tunnel: w269 -> [w324 _]
          frame False {
            n219 = call "File_setup.vi"("Measurement is top level?"=w324, "Results file"=w332, "Raw data file"=w330, "setup"=w329, "File"=w328) -> ("Results file output"=w331:path, "Raw data file output"=w325:path, "Raw data option"=w327:enum16{"Save raw data", "Raw data not saved"}, "File output"=w326:T13)
          }
          frame True {
            w336 = enum16{"Save raw data", "Raw data not saved"}."Raw data not saved"  # Raw data option
            n220 = global read "Meas_global.vi" "Raw data option"() -> (w337:enum16{"Save raw data", "Raw data not saved"})
            n221 = Compound Arithmetic op=AND(w335, invert w334) -> (w333:bool)
            n222 = Select(t=w337, s=w333, f=w336) -> (s? t:f=w338:enum16{"Save raw data", "Raw data not saved"})
          }
        }
        n223 = case shown="\"Save raw data\"" w272 {
          tunnel: w280 -> [w321 w323]
          tunnel: [w321 w322] -> w279
          frame "Raw data not saved" {
          }
          frame "Save raw data" {
            n224 = call "Find_Unique_Filename.vi"("Path In"=w323) -> ("Unique Path Out"=w322:path)  [unwired: 1 in, 1 out]
          }
        }
        n225 = local write "Results file"(w291) -> ()
        n226 = global write "Meas_global.vi" "Results file"(w291) -> ()
        n227 = global write "Meas_global.vi" "Raw data option"(w272) -> ()
        n228 = global write "Meas_global.vi" "File"(w278) -> ()
        n229 = global write "Meas_global.vi" "Raw data file"(w279) -> ()
        n230 = local write "Raw data file"(w279) -> ()
        n231 = local write "File"(w283) -> ()
      }
      frame #10 {
        n232 = global read "Meas_global.vi" "Ch & spans"() -> (w342:T28[])
        n233 = local read "Block average display control"() -> (w346:cluster{"Name":string, "Include":bool}[])
        n234 = global read "Meas_global.vi" "Analysis Info cluster"() -> (w343:T22[])
        n235 = for {
          tunnel: w343 -> [w354] mode=indexing
          tunnel: w346 -> [w353]
          tunnel: [w349] -> w345 mode=indexing
          tunnel: [w350] -> w344 mode=indexing
          i -> [w352]
          n236 = Unbundle By Name(w354) -> ("Symbol"=w349:string)
          n237 = Index Array(array=w353, index=w352) -> (element=w351:cluster{"Name":string, "Include":bool})
          n238 = Bundle By Name(cluster=w351, "Name"=w349) -> (w350:cluster{"Name":string, "Include":bool})
        }
        n239 = global write "Meas_global.vi" "Ch & spans + mod limits"(w342) -> ()
        n240 = local write "Block average display control"(w344) -> ()
        n241 = Build Array (concatenate)("Nothing", w345) -> (w347:string[])
        n242 = property on="Plot 1" class="Ring (strict)"("Strings []"=w347) -> ()  [unwired: 2 in, 2 out]
        n243 = property on="Plot 1" class="Ring (strict)"("Strings []"=w347) -> ()  [unwired: 2 in, 2 out]
        n244 = property on="Plot 2" class="Ring (strict)"("Strings []"=w347) -> ()  [unwired: 2 in, 2 out]
        n245 = property on="Plot 2" class="Ring (strict)"("Strings []"=w347) -> ()  [unwired: 2 in, 2 out]
      }
      frame #11 {
        n246 = global read "Meas_global.vi" "Analysis Info cluster"() -> (w357:T22[])
        n247 = for {
          tunnel: w357 -> [w478] mode=indexing
          tunnel: [w477] -> w358
          stop <- w477 stop-if-true
          n248 = Unbundle By Name(w478) -> ("Inst type"=w479:T16)
          n249 = Equal?(x=w479, y=Inst_type."LDA Vel" ("Inst type")) -> (x = y?=w477:bool)
        }
        n250 = global read "Meas_global.vi" "Post Process"() -> (w361:T2)
        n251 = Equal?(x=w361, y=Post_Process."Post Process Raw Data File" ("Post Process")) -> (x = y?=w359:bool)
        n252 = And(x=w358, y=w359) -> (x .and. y?=w355:bool)
        n253 = stacked-sequence {
          seq-local: [w363 _ _ _] -> [_ w391 w447 _]
          seq-local: [_ w393 _ _] -> [_ _ w446 _]
          seq-local: [w362 _ _ _] -> [_ w390 _ _]
          tunnel: w357 -> [w366 w394 _ w476]
          tunnel: w355 -> [_ w395 _ _]
          tunnel: "Correlate?" -> [_ w392 _ _]
          frame #0 {
            w364 = "RV (WT"
            n254 = String Length(string=w364) -> (length=w365:i32)
            n255 = for {
              tunnel: w366 -> [w385] mode=indexing
              shift-right: [w375] -> w367
              shift-left: i32[] [] -> [w376]
              tunnel: w365 -> [w373]
              tunnel: w364 -> [w371]
              tunnel: [w369] -> w362 mode=indexing
              i -> [w377]
              n256 = Unbundle By Name(w385) -> ("Inst name"=w369:string, "Symbol"=w384:string, "Code name"=w382:string)
              n257 = String Subset(string=w369, length (rest)=w373) -> (substring=w372:string)  [unwired: 1 in]
              n258 = Match Pattern(string=w382, regular expression="Derived") -> (offset past match=w381:i32)  [unwired: 1 in, 3 out]
              n259 = Not Equal?(x=w371, y=w372) -> (x != y?=w370:bool)
              n260 = Less Than 0?(x=w381) -> (x < 0?=w380:bool)
              n261 = Not Equal?(x="Sync", y=w384) -> (x != y?=w379:bool)
              n262 = Compound Arithmetic op=AND(w370, w379, w380) -> (w378:bool)
              n263 = case shown="True" w378 {
                tunnel: w377 -> [_ w389]
                tunnel: w376 -> [w386 w388]
                tunnel: [w386 w387] -> w375
                frame False {
                }
                frame True {
                  n264 = Build Array (concatenate)(w388, w389) -> (w387:i32[])
                }
              }
            }
            n265 = call "Chs_to_Correlate.vi"("Valid Ch to correlate"=w367) -> ("Correlation Pairs"=w363:i32[][])
          }
          frame #1 {
            n266 = case shown="False" w395 {
              tunnel: w394 -> [_ _]
              tunnel: [w396 w443] -> w393
              tunnel: w392 -> [w402 _]
              tunnel: w391 -> [w397 w443]
              tunnel: w390 -> [w403 _]
              frame False {
                n267 = global read "Meas_global.vi" "correlate"() -> (w400:i32[][])
                n268 = for {
                  tunnel: w397 -> [w428] mode=indexing
                  tunnel: w403 -> [w433]
                  tunnel: [w424] -> w401 mode=indexing
                  tunnel: w400 -> [w429]
                  shift-right: [w425] -> w398
                  shift-left: string[] [] -> [w426]
                  n269 = Index Array(array=w428) -> (element #1=w435:i32, element #2=w434:i32)  [unwired: 2 in]
                  n270 = for {
                    tunnel: w428 -> [w442]
                    tunnel: w429 -> [w441] mode=indexing
                    tunnel: [w440] -> w427
                    stop <- w440 stop-if-true
                    n271 = Equal?(x=w442, y=w441) -> (x = y?=w440:bool)
                  }
                  n272 = Index Array(array=w433, index=w435) -> (element=w432:string)
                  n273 = Index Array(array=w433, index=w434) -> (element=w431:string)
                  n274 = Format Into String(format string="%s & %s", w432, w431) -> (resulting string=w424:string)  [unwired: 2 in, 1 out]
                  n275 = case shown="True" w427 {
                    tunnel: w426 -> [w436 w439]
                    tunnel: [w436 w438] -> w425
                    tunnel: w424 -> [_ w437]
                    frame False {
                    }
                    frame True {
                      n276 = Build Array (concatenate)(w439, w437) -> (w438:string[])
                    }
                  }
                }
                n277 = case shown="\"Correlate without activating panel\"" w402 {
                  tunnel: w401 -> [_ w411 w415]
                  tunnel: w398 -> [_ w409 w416]
                  tunnel: w397 -> [_ w407 w417]
                  tunnel: [i32[][] [] ("Correlation Pairs") w405 w418] -> w396
                  frame "Cross correlation off" {
                  }
                  frame "Show correlation panel" {
                    n278 = call "Select_Strings.vi"("Available Ch names"=w411, "Message"="Please select Channels to Correlate", "Selector mode"=T14."Zero or more", "Desired Ch names (in)"=w409) -> ("Ch Indicies Choosen"=w406:i32[])  [unwired: 2 in, 2 out]
                    n279 = for {
                      tunnel: w407 -> [w414]
                      tunnel: w406 -> [w413] mode=indexing
                      tunnel: [w412] -> w405 mode=indexing
                      n280 = Index Array(array=w414, index (row)=w413) -> (element=w412:i32[])  [unwired: 1 in]
                    }
                  }
                  frame "Correlate without activating panel" {
                    n281 = for {
                      tunnel: [w423] -> w418 mode=indexing
                      tunnel: w417 -> [w422]
                      tunnel: w416 -> [w421] mode=indexing
                      tunnel: w415 -> [w420]
                      n282 = Search 1D Array(1D array=w420, element=w421) -> (index of element=w419:i32)  [unwired: 1 in]
                      n283 = Index Array(array=w422, index (row)=w419) -> (element=w423:i32[])  [unwired: 1 in]
                    }
                  }
                }
              }
              frame True {
              }
            }
          }
          frame #2 {
            n284 = for {
              shift-right: [w454] -> w444
              shift-left: i32[][] [] -> [w455]
              tunnel: w447 -> [w456]
              tunnel: w446 -> [w453] mode=indexing
              n285 = for {
                tunnel: w456 -> [w471] mode=indexing
                tunnel: w453 -> [w470]
                tunnel: [w469] -> w452
                stop <- w469 stop-if-true
                n286 = Equal?(x=w470, y=w471) -> (x = y?=w469:bool)
              }
              n287 = case shown="True" w452 {
                tunnel: w455 -> [w457 w459]
                tunnel: w453 -> [_ w460]
                tunnel: [w457 w461] -> w454
                frame False {
                }
                frame True {
                  n288 = for {
                    tunnel: w460 -> [w464]
                    tunnel: w459 -> [w463] mode=indexing
                    tunnel: [w462] -> w458
                    stop <- w462 stop-if-true
                    n289 = Equal?(x=w464, y=w463) -> (x = y?=w462:bool)
                  }
                  n290 = case shown="False" w458 {
                    tunnel: w459 -> [w467 w468]
                    tunnel: w460 -> [w466 _]
                    tunnel: [w465 w468] -> w461
                    frame False {
                      n291 = Build Array (concatenate)(w467, w466) -> (w465:i32[][])
                    }
                    frame True {
                    }
                  }
                }
              }
            }
            n292 = global write "Meas_global.vi" "correlate"(w444) -> ()
            n293 = Array Size(array=w444) -> (size(s)=w451:i32[])
            n294 = Index Array(array=w451, index=0) -> (element=w448:i32)
            n295 = Equal To 0?(x=w448) -> (x = 0?=w449:bool)
            n296 = case shown="True" w449 {
              frame False {
              }
              frame True {
                n297 = local write "Correlate?"(T9."Cross correlation off" ("Correlate?")) -> ()
              }
            }
          }
          frame #3 {
            n298 = Array Size(array=w476) -> (size(s)=w474:i32)
            n299 = Initialize Array(T15 {"Weighting"=[], "Time (ms)"=[], "Voltage"=[], "Eng Values"=[]} ("Time Trace"), w474) -> (w473:T29)
            n300 = global write "Meas_global.vi" "Time Trace"(w473) -> ()
          }
        }
      }
      frame #12 {
        n301 = stacked-sequence {
          seq-local: [w487 _] -> [_ w509]
          tunnel: w481 -> [w486 _]
          frame #0 {
            n302 = call "LDA+_An_Analysis_mode.vi"("Second Graph"="Second Graph", "First Graph"="First Graph") -> ("Second Graph out"=w482:T8, "First Graph out"=w484:T8)  [unwired: 6 out]
            n303 = case shown="False" w486 {
              tunnel: [w497 w508] -> w485
              tunnel: w484 -> [w496 w508]
              tunnel: [w495 w507] -> w483
              tunnel: w482 -> [w494 w507]
              frame False {
                w492 = Graph_Type."Show no graph" ("Plot Type")
                n304 = Unbundle By Name(w496) -> ("Save graph"=w498:u16)
                n305 = Unbundle By Name(w494) -> ("Save graph"=w493:u16)
                n306 = case shown="0, Default" w498 {
                  tunnel: [w504 w506] -> w497
                  tunnel: w496 -> [w505 w506]
                  tunnel: w492 -> [w503 _]
                  frame 0, Default {
                    n307 = Bundle By Name(cluster=w505, "Plot Type"=w503) -> (w504:T8)
                  }
                  frame 1 {
                  }
                }
                n308 = case shown="0, Default" w493 {
                  tunnel: [w500 w502] -> w495
                  tunnel: w494 -> [w501 w502]
                  tunnel: w492 -> [w499 _]
                  frame 0, Default {
                    n309 = Bundle By Name(cluster=w501, "Plot Type"=w499) -> (w500:T8)
                  }
                  frame 1 {
                  }
                }
              }
              frame True {
              }
            }
            n310 = local write "Second Graph"(w483) -> ()
            n311 = local write "First Graph"(w485) -> ()
            n312 = global write "Meas_global.vi" "Second Graph"(w483) -> ()
            n313 = global write "Meas_global.vi" "First Graph"(w485) -> ()
            n314 = Unbundle By Name(w483) -> ("Plot Type"=w491:T7)
            n315 = Unbundle By Name(w485) -> ("Plot Type"=w490:T7)
            n316 = Build Array(w490, w491) -> (w487:T7[])
          }
          frame #1 {
            n317 = global read "Meas_global.vi" "Insts for plotting"() -> (w510:u16[][])
            n318 = for {
              tunnel: w510 -> [w512] mode=indexing
              tunnel: w509 -> [w511] mode=indexing
              i -> [w513]
              n319 = stacked-sequence {
                seq-local: [w516 _] -> [_ w528]
                seq-local: [w517 _] -> [_ w527]
                tunnel: w513 -> [_ w531]
                tunnel: w512 -> [w515 _]
                tunnel: w511 -> [_ w523]
                frame #0 {
                  n320 = property on="Plot 1" class="Ring (strict)"() -> ("Strings []"=w514:string[])  [unwired: 2 in, 2 out]
                  n321 = Array To Cluster(array=w515) -> (cluster=w520:T30)
                  n322 = Unbundle(w520) -> ("Insts for plotting[0]"=w519:u16, "Insts for plotting[1]"=w518:u16)
                  n323 = Index Array(array=w514, index=w519) -> (element=w516:string)
                  n324 = Index Array(array=w514, index=w518) -> (element=w517:string)
                }
                frame #1 {
                  n325 = case shown="\"Show no graph\"" w523 {
                    tunnel: [u8 0 u8 0 u8 0 u8 0 u8 0 u8 1 u8 0] -> w535
                    tunnel: [u8 0 u8 0 u8 0 u8 0 u8 1 u8 1 u8 0] -> w534
                    tunnel: [u8 0 u8 0 u8 0 u8 0 u8 1 u8 1 u8 0] -> w533
                    tunnel: [u8 0 u8 0 u8 0 u8 0 u8 1 u8 0 u8 0] -> w532
                    tunnel: [FALSE TRUE TRUE TRUE TRUE TRUE TRUE] -> w526
                    tunnel: [u8 0 u8 1 u8 1 u8 2 u8 0 u8 0 u8 2] -> w525
                    tunnel: [u8 0 u8 4 u8 1 u8 2 u8 0 u8 0 u8 1] -> w524
                    tunnel: ["" "Time (s)" "Time (s)" "" "" "" ""] -> w522
                    tunnel: ["" "Voltage" "Velocity" "" "" "" ""] -> w521
                    frame "Show no graph" {
                    }
                    frame "Voltage trace" {
                    }
                    frame "Velocity trace" {
                    }
                    frame "Vel histogram" {
                    }
                    frame "Spectrum" {
                    }
                    frame "f.E(f) v Log f" {
                    }
                    frame "Auto-Corr" {
                    }
                  }
                  n326 = case shown="0, Default" w531 {
                    tunnel: w526 -> [w548 w561]
                    tunnel: w535 -> [w547 w560]
                    tunnel: w534 -> [w546 w559]
                    tunnel: w533 -> [w545 w558]
                    tunnel: w532 -> [w544 w557]
                    tunnel: u32 0 -> [w543 w556]
                    tunnel: u32 1 -> [w542 w554]
                    tunnel: w528 -> [w541 w555]
                    tunnel: w527 -> [w540 w553]
                    tunnel: w525 -> [w539 w552]
                    tunnel: w524 -> [w538 w551]
                    tunnel: w522 -> [w537 w550]
                    tunnel: w521 -> [w536 w549]
                    frame 0, Default {
                      n327 = property on="First plot" class="XYGraph (strict)"("Visible"=w548, "X Scale.Format & Precision:Format"=w547, "X Scale.Mapping Mode"=w546, "Y Scale.Format & Precision:Format"=w545, "Y Scale.Mapping Mode"=w544, "Active Plot"=w543, "Plot.Plot Name"=w541, "Active Plot"=w542, "Plot.Plot Name"=w540, "X Scale.Format & Precision:Precision"=w539, "Y Scale.Format & Precision:Precision"=w538, "XScale.NameLbl.Text"=w537, "YScale.NameLbl.Text"=w536) -> ()  [unwired: 2 in, 2 out]
                    }
                    frame 1 {
                      n328 = property on="2nd plot" class="XYGraph (strict)"("Visible"=w561, "X Scale.Format & Precision:Format"=w560, "X Scale.Mapping Mode"=w559, "Y Scale.Format & Precision:Format"=w558, "Y Scale.Mapping Mode"=w557, "Active Plot"=w556, "Plot.Plot Name"=w555, "Active Plot"=w554, "Plot.Plot Name"=w553, "X Scale.Format & Precision:Precision"=w552, "Y Scale.Format & Precision:Precision"=w551, "XScale.NameLbl.Text"=w550, "YScale.NameLbl.Text"=w549) -> ()  [unwired: 2 in, 2 out]
                    }
                  }
                }
              }
            }
          }
        }
      }
      frame #13 {
        n329 = local read "Second Graph"() -> (w636:T8)
        n330 = local read "First Graph"() -> (w635:T8)
        n331 = Unbundle By Name(w635) -> ("Plot 1"=w628:u16, "Plot 2"=w629:u16)
        n332 = Unbundle By Name(w636) -> ("Plot 1"=w630:u16, "Plot 2"=w631:u16)
        n333 = Build Array(w628, w629) -> (w632:u16[])
        n334 = Build Array(w630, w631) -> (w633:u16[])
        n335 = global read "Meas_global.vi" "Analysis Info cluster"() -> (w637:T22[])
        n336 = Decrement(x=w632) -> (x-1=w626:u16[])
        n337 = Decrement(x=w633) -> (x-1=w634:u16[])
        n338 = for {
          tunnel: w637 -> [w645]
          tunnel: w626 -> [w644] mode=indexing
          shift-right: [w638] -> _
          shift-left: u32 0 -> [w640]
          i -> [w639]
          n339 = Index Array(array=w645, index=w644) -> (element=w646:T22)
          n340 = Unbundle By Name(w646) -> ("Colour"=w641:u32)
          n341 = Equal?(x=w641, y=w640) -> (x = y?=w643:bool)
          n342 = Select(t=u32 13434624, s=w643, f=w641) -> (s? t:f=w638:u32)
          n343 = property on="First plot" class="XYGraph (strict)"("Active Plot"=w639, "Plot.Plot Color"=w638, "Plot.Fill/Point Color"=w638) -> ()  [unwired: 2 in, 2 out]
        }
        n344 = for {
          tunnel: w637 -> [w654]
          tunnel: w634 -> [w653] mode=indexing
          shift-right: [w649] -> _
          shift-left: u32 0 -> [w647]
          i -> [w652]
          n345 = Index Array(array=w654, index=w653) -> (element=w655:T22)
          n346 = Unbundle By Name(w655) -> ("Colour"=w648:u32)
          n347 = Equal?(x=w648, y=w647) -> (x = y?=w651:bool)
          n348 = Select(t=u32 13434624, s=w651, f=w648) -> (s? t:f=w649:u32)
          n349 = property on="2nd plot" class="XYGraph (strict)"("Active Plot"=w652, "Plot.Plot Color"=w649, "Plot.Fill/Point Color"=w649) -> ()  [unwired: 2 in, 2 out]
        }
      }
      frame #14 {
        n350 = global read "DataTranslation_global.vi" "Different Sampling Freq per block"() -> (w656:bool)
        n351 = global read "Meas_global.vi" "Remote control"() -> (w665:bool)
        n352 = global read "Meas_global.vi" "Post Process"() -> (w668:T2)
        n353 = global read "Meas_global.vi" "PWA Data"() -> (w657:T31)
        n354 = case shown="\"No PWA Data\"" w657 {
          tunnel: [w669 w674] -> w659
          frame "No PWA Data" {
            n355 = local read "Desired Sampling freq (Hz)"() -> (w671:dbl)
            n356 = local read "No of samples"() -> (w670:i32)
            n357 = Divide(x=w670, y=w671) -> (x/y=w669:dbl)
          }
          frame "One Ch PWA" {
            n358 = local read "No of samples"() -> (w672:i32)
            n359 = global read "PWAtasksGLOBAL.vi" "PWA Freq. (Hz)"() -> (w673:dbl)
            n360 = global write "PWAtasksGLOBAL.vi" "PWA No. of Samples"(w672) -> ()
            n361 = Divide(x=w672, y=w673) -> (x/y=w674:dbl)
          }
        }
        n362 = global read "Meas_global.vi" "Averaging time (min)"() -> (w663:dbl)
        n363 = Equal?(x=Setup."Run Program" ("setup"), y=w662) -> (x = y?=w660:bool)
        n364 = Equal?(x=Post_Process."Take New Data" ("Post Process"), y=w668) -> (x = y?=w664:bool)
        n365 = Compound Arithmetic op=AND(invert w656, w664, invert w658, invert w665, w660) -> (w666:bool)
        n366 = case shown="True" w666 {
          tunnel: w663 -> [_ w681]
          tunnel: w659 -> [_ w680]
          frame False {
          }
          frame True {
            n367 = Multiply(x=w681, y=60.0) -> (x*y=w677:dbl)
            n368 = Divide(x=w677, y=w680) -> (x/y=w676:dbl)
            n369 = Round Toward +Infinity(x=w676) -> (ceil(x): smallest int >= x=w675:dbl)
            n370 = To Long Integer(number=w675) -> (32bit integer=w679:i32)
            n371 = global write "Meas_global.vi" "Requested No of blocks"(w679) -> ()
            n372 = local write "No of Blocks"(w679) -> ()
          }
        }
      }
      frame #15 {
        n373 = case shown="\"Run Program\"" w682 {
          frame "Run Program" {
            n374 = call "Read_calibration_files.vi"() -> ()  [unwired: 1 out]
            n375 = global write "Meas_global.vi" "Repeat Measurement?"(FALSE ("Repeat Measurement?")) -> ()
          }
          frame "Show Setup", Default {
          }
        }
      }
      frame #16 {
        n376 = global read "Meas_global.vi" "Raw data option"() -> (w687:enum16{"Save raw data", "Raw data not saved"})
        n377 = Get Date/Time In Seconds() -> (seconds since 1Jan1904=w688:timestamp)
        n378 = To Double Precision Float(number=w688) -> (double precision float=w685:dbl)
        n379 = global read "Meas_global.vi" "Post Process"() -> (w686:T2)
        n380 = case shown="\"Setup Front Panel\"" w689 {
          tunnel: w687 -> [w691 _ _ _]
          tunnel: w686 -> [w690 _ w732 w741]
          frame "Run Program" {
            n381 = case shown="\"Take New Data\"" w690 {
              tunnel: w691 -> [w701 _]
              frame "Take New Data" {
                n382 = case shown="\"Save raw data\"" w701 {
                  frame "Save raw data" {
                  }
                  frame "Raw data not saved" {
                    w709 = FALSE  # Lock File
                    w706 = FALSE  # advisory dialog? (display:T)
                    w705 = FALSE  # append to file? (new file:F)
                    n383 = global read "Meas_global.vi" "Remote control"() -> (w707:bool)
                    n384 = call "Create_setup_string.vi"() -> ("Setup String"=w710:string)  [unwired: 1 out]
                    n385 = case shown="False" w707 {
                      tunnel: ["Current_Setup.xls" ("Setup filename") w712] -> w702
                      frame False {
                      }
                      frame True {
                        n386 = local read "Setup filename"() -> (w712:string)
                      }
                    }
                    n387 = call "Add_length_to_string.vi"("String in"=w710) -> ("String out"=w708:string)
                    n388 = call "Setup_Filepath.vi"("Setup File Type"=Setup_Filetype."Measurement Setups", "Filename in"=w702) -> ("Filename Out"=w703:path)  [unwired: 1 out]
                    n389 = call "Write_Characters_To_File.vi"("file path (dialog if empty)"=w703, "advisory dialog? (display:T)"=w706, "character string"=w708, "append to file? (new file:F)"=w705, "Lock File"=w709) -> ()  [unwired: 4 out]
                  }
                }
                n390 = global read "Meas_global.vi" "Requested No of samples"() -> (w695:i32)
                n391 = global read "Meas_global.vi" "Requested Sampling rate"() -> (w698:dbl)
                n392 = global read "Meas_global.vi" "Requested No of blocks"() -> (w694:i32)
                n393 = Divide(x=w695, y=w698) -> (x/y=w697:dbl)
                n394 = Multiply(x=w694, y=w697) -> (x*y=w693:dbl)
                n395 = Add(x=w693, y=120.0) -> (x+y=w692:dbl)
                n396 = call "Program_Active_Client.vi"("Mode"=enum16{"Program Active", "Traverse Level State"}."Program Active", "Time till next contact (Sec)"=w692, "Traverse level State"=Traverse_Level_State."Running") -> ()  [unwired: 3 out]
              }
              frame "Post Process Raw Data File" {
              }
            }
          }
          frame "Save Current Setup" {
            n397 = stacked-sequence {
              seq-local: [w715 _] -> [_ w718]
              seq-local: [w714 _] -> [_ w717]
              frame #0 {
                w716 = FALSE  # Save New File?
                n398 = call "Save_current_setup.vi"("Save New File?"=w716, "Setup File Type"=Setup_Filetype."Measurement Setups") -> ("Cancelled?"=w714:bool, "Saved filepath"=w715:path)  [unwired: 2 out]
              }
              frame #1 {
                n399 = case shown="False" w717 {
                  tunnel: w718 -> [w724 _]
                  frame False {
                    w721 = "Initial Probe positions" ("File Label")
                    w729 = FALSE  # append to file? (new file:F)
                    w730 = FALSE  # advisory dialog? (display:T)
                    w731 = FALSE  # Lock File
                    n400 = call "Input_Instrument_Positions.vi"("Filepath to Save"=w724) -> ("Output string"=w723:string)  [unwired: 1 out]
                    n401 = call "Create_setup_string.vi"() -> ("Setup String"=w722:string)  [unwired: 1 out]
                    n402 = call "Get_string_subset.vi"("String to split"=w723, "File Label"=w721) -> ("Output string"=w720:string)  [unwired: 2 in, 1 out]
                    n403 = call "Replace_data_in_Label_str.vi"("New data string"=w720, "Input string"=w722, "Variable name"=w721) -> ("Appended string"=w719:string)
                    n404 = call "Replace_data_in_setup_string.vi"("New data string"="", "Input string"=w719, "Variable name"="Comments") -> ("Appended string"=w725:string)
                    n405 = call "Add_length_to_string.vi"("String in"=w725) -> ("String out"=w728:string)
                    n406 = call "Write_Characters_To_File.vi"("file path (dialog if empty)"=w724, "advisory dialog? (display:T)"=w730, "character string"=w728, "append to file? (new file:F)"=w729, "Lock File"=w731) -> ()  [unwired: 4 out]
                  }
                  frame True {
                  }
                }
              }
            }
          }
          frame "Show Setup" {
            n407 = case shown="\"Take New Data\"" w732 {
              frame "Take New Data" {
                w737 = FALSE  # append to file? (new file:F)
                w738 = FALSE  # advisory dialog? (display:T)
                w739 = FALSE  # Lock File
                n408 = call "Create_setup_string.vi"() -> ("Setup String"=w740:string)  [unwired: 1 out]
                n409 = call "Add_length_to_string.vi"("String in"=w740) -> ("String out"=w736:string)
                n410 = call "Setup_Filepath.vi"("Setup File Type"=Setup_Filetype."Measurement Setups", "Filename in"="Current_Setup.xls" ("Setup filename")) -> ("Filename Out"=w734:path)  [unwired: 1 out]
                n411 = call "Write_Characters_To_File.vi"("file path (dialog if empty)"=w734, "advisory dialog? (display:T)"=w738, "character string"=w736, "append to file? (new file:F)"=w737, "Lock File"=w739) -> ()  [unwired: 4 out]
              }
              frame "Post Process Raw Data File" {
              }
            }
          }
          frame "Setup Front Panel" {
            n412 = case shown="\"Take New Data\"" w741 {
              frame "Take New Data" {
                w746 = FALSE  # append to file? (new file:F)
                w747 = FALSE  # advisory dialog? (display:T)
                w748 = FALSE  # Lock File
                n413 = call "Create_setup_string.vi"() -> ("Setup String"=w749:string)  [unwired: 1 out]
                n414 = call "Add_length_to_string.vi"("String in"=w749) -> ("String out"=w745:string)
                n415 = call "Setup_Filepath.vi"("Setup File Type"=Setup_Filetype."Measurement Setups", "Filename in"="Current_Setup.xls" ("Setup filename")) -> ("Filename Out"=w743:path)  [unwired: 1 out]
                n416 = call "Write_Characters_To_File.vi"("file path (dialog if empty)"=w743, "advisory dialog? (display:T)"=w747, "character string"=w745, "append to file? (new file:F)"=w746, "Lock File"=w748) -> ()  [unwired: 4 out]
              }
              frame "Post Process Raw Data File" {
              }
            }
          }
        }
        n417 = global write "Meas_global.vi" "Actual Measurement time (min)"(0.0 ("Max Measurement time (min)")) -> ()
      }
      frame #17 {
        n418 = case shown="\"Setup Front Panel\", Default" w753 {
          tunnel: w750 -> [w755 _]
          tunnel: w752 -> [_ w848]
          tunnel: w751 -> [w754 _]
          frame "Run Program" {
            n419 = while {
              tunnel: w755 -> [w757]
              tunnel: w754 -> [w756]
              i -> [w758]
              stop <- w759 stop-if-true
              n420 = Increment(x=w758) -> (x+1=w760:i32)
              n421 = stacked-sequence {
                seq-local: [_ _ _ _ _ "Block average display control" _ _ _ _] -> [_ _ _ _ _ _ w793 _ _ _]
                seq-local: [_ _ _ _ _ _ w791 _ _ _] -> [_ _ _ _ _ _ _ w809 _ _]
                seq-local: [_ _ _ _ w774 _ _ _ _ _] -> [_ _ _ _ _ _ _ _ _ w841]
                seq-local: [_ w762 _ _ _ _ _ _ _ _] -> [_ _ w766 _ _ _ _ _ _ _]
                seq-local: [_ _ w764 _ _ _ _ _ _ _] -> [_ _ _ _ _ _ _ _ _ w844]
                tunnel: w760 -> [w761 _ w765 _ _ w783 _ _ _ w845]
                tunnel: [_ _ w764 _ _ _ _ _ _ _] -> w759
                tunnel: w757 -> [_ _ _ _ w773 _ _ _ _ _]
                tunnel: w756 -> [_ _ _ _ _ _ _ _ _ _]
                frame #0 {
                  n422 = global write "Meas_global.vi" "Current Block No"(w761) -> ()
                  "Current Block No" <- w761
                }
                frame #1 {
                  n423 = call "Get_data.vi"() -> ("EOF? and Error status"=w762:bool, "Block Header"=w763:string)  [unwired: 10 out]
                  n424 = global write "Plug_in_data_global.vi" "Block Header"(w763) -> ()
                }
                frame #2 {
                  w768 = string[] [] ("Plug in titles")
                  n425 = global write "Meas_global.vi" "Requested No of blocks"("No of Blocks") -> ()
                  n426 = Less Or Equal?(x="No of Blocks", y=w765) -> (x <= y?=w769:bool)
                  n427 = Compound Arithmetic op=OR(w766, w769) -> (w764:bool)
                  n428 = case shown="True" w764 {
                    tunnel: w765 -> [_ w770]
                    frame False {
                    }
                    frame True {
                      n429 = global write "Meas_global.vi" "Requested No of blocks"(w770) -> ()
                      n430 = local write "No of Blocks"(w770) -> ()
                    }
                  }
                  n431 = global write "Meas_global.vi" "Processing last block?"(w764) -> ()
                  n432 = global write "Dynamic_call_global.ph.vi" "Plug in values"(w768) -> ()
                  n433 = global write "Dynamic_call_global.ph.vi" "Plug in titles"(w768) -> ()
                  n434 = global write "PWAtasksGLOBAL.vi" "STOP"(w764) -> ()
                }
                frame #3 {
                  n435 = call "Text_without_format.vi"("Input string"="Comments") -> ("Output string"=w771:string)
                  n436 = local write "Comments"(w771) -> ()
                  n437 = global write "Meas_global.vi" "Comments"(w771) -> ()
                }
                frame #4 {
                  n438 = call "Process_data.vi"("Measurement top level?"=w773) -> ("Vel stat display"=→"Statistics":string[][], "First Plot data Cluster"=→"First plot":cluster{"X array":dbl[], "Y array":dbl[]}[], "Second Plot Data Cluster"=→"2nd plot":cluster{"X array":dbl[], "Y array":dbl[]}[], "Max Measurement time up"=w774:bool)  [unwired: 5 in]
                }
                frame #5 {
                  n439 = global read "Meas_global.vi" "Actual Measurement time (min)"() -> (→"Measurement time (min)":dbl)
                  n440 = global read "Meas_global.vi" "Actual Sampling rate (Hz)"() -> (→"Actual Sampling freq":dbl)
                  n441 = call "Display_blocks.vi"("Block No"=w783, "Block average display"="Block average display control") -> ("u^4"=→"u^4":dbl[][], "u^3"=→"u^3":dbl[][], "uv"=→"uv":dbl[][], "u^2"=→"u^2" →"Array u^2":dbl[][], "U"=→"U" →"Array U":dbl[][])  [unwired: 4 out]
                }
                frame #6 {
                  n442 = global read "Meas_global.vi" "Analysis Info cluster"() -> (w792:T22[])
                  n443 = global read "Meas_global.vi" "Diagnostic info"() -> (w790:string[][])
                  n444 = for {
                    tunnel: w793 -> [w808] mode=indexing
                    tunnel: w792 -> [w805] mode=indexing
                    tunnel: [w807] -> w791 mode=indexing if=w806
                    tunnel: [w795] -> w789 mode=indexing
                    tunnel: [w794] -> w788 mode=indexing
                    n445 = Unbundle By Name(w805) -> ("Colour"=w807:u32)
                    n446 = Unbundle By Name(w808) -> ("Include"=w806:bool)
                    n447 = Unbundle By Name(w805) -> ("Inst name"=w799:string, "Av Sampling Rate"=w801:dbl, "Av No of Samples"=w798:dbl)
                    n448 = Format Into String(format string="%s Freq Hz", w799) -> (resulting string=w803:string)  [unwired: 2 in, 1 out]
                    n449 = Format Into String(format string="%s Samples per block", w799) -> (resulting string=w796:string)  [unwired: 2 in, 1 out]
                    n450 = Number To Decimal String(number=w801) -> (decimal integer string=w802:string)  [unwired: 1 in]
                    n451 = Number To Decimal String(number=w798) -> (decimal integer string=w797:string)  [unwired: 1 in]
                    n452 = Build Array(w803, w802) -> (w795:string[])
                    n453 = Build Array(w796, w797) -> (w794:string[])
                  }
                  n454 = Build Array (concatenate)(w790, w789, w788) -> (→"Diagnostic info":string[][])
                }
                frame #7 {
                  n455 = for {
                    tunnel: w809 -> [w810] mode=indexing
                    i -> [w811]
                    n456 = property on="U" class="WFGraph (strict)"("Active Plot"=w811, "Plot.Plot Color"=w810, "Plot.Fill/Point Color"=w810) -> ()  [unwired: 2 in, 2 out]
                    n457 = property on="u^3" class="WFGraph (strict)"("Active Plot"=w811, "Plot.Plot Color"=w810, "Plot.Fill/Point Color"=w810) -> ()  [unwired: 2 in, 2 out]
                    n458 = property on="u^4" class="WFGraph (strict)"("Active Plot"=w811, "Plot.Plot Color"=w810, "Plot.Fill/Point Color"=w810) -> ()  [unwired: 2 in, 2 out]
                    n459 = property on="u^2" class="WFGraph (strict)"("Active Plot"=w811, "Plot.Plot Color"=w810, "Plot.Fill/Point Color"=w810) -> ()  [unwired: 2 in, 2 out]
                  }
                }
                frame #8 {
                  n460 = case shown="True" "Pause" {
                    frame False {
                    }
                    frame True {
                      n461 = global read "Meas_global.vi" "Post Process"() -> (w813:T2)
                      n462 = case shown="\"Take New Data\"" w813 {
                        frame "Take New Data" {
                          n463 = call "Program_Active_Client.vi"("Mode"=enum16{"Program Active", "Traverse Level State"}."Program Active", "Time till next contact (Sec)"=12000.0, "Traverse level State"=Traverse_Level_State."Running") -> ()  [unwired: 3 out]
                          n464 = while {
                            i -> [w820]
                            stop <- w821 continue-if-true
                            n465 = Quotient & Remainder(x=w820, y=10) -> (x-y*floor(x/y)=w818:i32)  [unwired: 1 out]
                            n466 = Equal To 0?(x=w818) -> (x = 0?=w817:bool)
                            n467 = stacked-sequence {
                              seq-local: [_ w823 _ _] -> [_ _ w825 _]
                              tunnel: [_ w823 _ _] -> w821
                              tunnel: w817 -> [_ _ _ w827]
                              frame #0 {
                                "Pause message" <- "Measurement Program Paused!!!!" ("Pause message")
                              }
                              frame #1 {
                                n468 = global write "Trav_pos_global.vi" "Paused During Row?"(TRUE ("Paused During Row?")) -> ()
                                n469 = local read "Pause"() -> (w823:bool)
                              }
                              frame #2 {
                                n470 = property on="Pause message" class="Str"("Blinking"=w825, "Visible"=w825) -> ()  [unwired: 2 in, 2 out]
                                n471 = Wait Until Next ms Multiple(millisecond multiple=u32 1000) -> ()  [unwired: 1 out]
                              }
                              frame #3 {
                                n472 = case shown="False" w827 {
                                frame False {
                                }
                                frame True {
                                n473 = Current VI's Path() -> (path=w828:path)
                                n474 = call "Bring_to_front.vi"("path"=w828) -> ()
                                }
                                }
                              }
                            }
                          }
                        }
                        frame "Post Process Raw Data File" {
                          n475 = stacked-sequence {
                            seq-local: [_ w831 _ _] -> [_ _ _ w838]
                            frame #0 {
                              n476 = property on="PP next block" class="Bool (strict)"("Visible"=TRUE) -> ()  [unwired: 2 in, 2 out]
                              n477 = local write "PP next block"(FALSE ("PP next block")) -> ()
                            }
                            frame #1 {
                              n478 = while {
                                tunnel: [w835] -> w831
                                stop <- w832 stop-if-true
                                n479 = local read "stop"() -> (w835:bool)
                                n480 = local read "Pause"() -> (w833:bool)
                                n481 = Compound Arithmetic op=OR(w835, "PP next block", invert w833) -> (w832:bool)
                                n482 = case shown="False" w832 {
                                frame False {
                                n483 = Wait (ms)(milliseconds to wait=u32 200) -> ()  [unwired: 1 out]
                                }
                                frame True {
                                }
                                }
                              }
                            }
                            frame #2 {
                              n484 = property on="PP next block" class="Bool (strict)"("Visible"=FALSE) -> ()  [unwired: 2 in, 2 out]
                            }
                            frame #3 {
                              n485 = Stop(stop? (T)=w838) -> ()
                            }
                          }
                        }
                      }
                    }
                  }
                }
                frame #9 {
                  n486 = global read "Meas_global.vi" "stop"() -> (w839:bool)
                  n487 = Compound Arithmetic op=OR("stop", w841, w839) -> (w840:bool)
                  n488 = Compound Arithmetic op=AND(w840, invert w844) -> (w843:bool)
                  n489 = case shown="True" w843 {
                    tunnel: w845 -> [_ w847]
                    frame False {
                    }
                    frame True {
                      n490 = Increment(x=w847) -> (x+1=w846:i32)
                      n491 = local write "No of Blocks"(w846) -> ()
                      n492 = global write "Meas_global.vi" "Requested No of blocks"(w846) -> ()
                    }
                  }
                }
              }
            }
          }
          frame "Setup Front Panel", Default {
            n493 = stacked-sequence {
              seq-local: [w849 _ _ _ _ _ _] -> [_ _ _ _ _ w929 _]
              seq-local: [_ w855 _ _ _ _ _] -> [_ _ _ _ _ w928 _]
              seq-local: [_ _ _ w887 _ _ _] -> [_ _ _ _ _ w927 _]
              seq-local: [_ _ _ _ w905 _ _] -> [_ _ _ _ _ w925 _]
              seq-local: [_ w854 _ _ _ _ _] -> [_ _ _ _ _ _ w938]
              seq-local: [_ _ w880 _ _ _ _] -> [_ _ _ _ _ w924 _]
              tunnel: w848 -> [_ w856 _ _ _ _ _]
              frame #0 {
                n494 = Build Array("Name", "Channel", "High limit", "Low limit") -> (w849:string[])
              }
              frame #1 {
                n495 = global read "Meas_global.vi" "LDA data"() -> (w854:enum16{"No LDA data", "Take LDA data"})
                n496 = case shown="\"Take LDA data\"" w854 {
                  tunnel: w856 -> [_ w867]
                  tunnel: [string[][] [] w864] -> w855
                  frame "No LDA data" {
                  }
                  frame "Take LDA data" {
                    n497 = global read "LDA_meas_global_1.vi" "Max Vel BSA1"() -> (w859:dbl)
                    n498 = global read "LDA_meas_global_1.vi" "Min Vel BSA1"() -> (w858:dbl)
                    n499 = global read "LDA_meas_global_1.vi" "Vel Comp BSA1"() -> (w868:string)
                    n500 = case shown="\"2D\"" w867 {
                      tunnel: [string[] [] w873] -> w865
                      frame "1D" {
                      }
                      frame "2D" {
                        n501 = global read "LDA_meas_global_2.vi" "Max Vel BSA2"() -> (w872:dbl)
                        n502 = global read "LDA_meas_global_2.vi" "Min Vel BSA2"() -> (w871:dbl)
                        n503 = global read "LDA_meas_global_2.vi" "Vel Comp BSA2"() -> (w874:string)
                        n504 = Format Into String(format string="%.1f m/s" ("Format String"), w871) -> (resulting string=w879:string)  [unwired: 2 in, 1 out]
                        n505 = Format Into String(format string="%.1f m/s" ("Format String"), w872) -> (resulting string=w878:string)  [unwired: 2 in, 1 out]
                        n506 = Build Array("LDA", w874, w878, w879) -> (w873:string[])
                      }
                    }
                    n507 = Format Into String(format string="%.1f m/s" ("Format String"), w858) -> (resulting string=w860:string)  [unwired: 2 in, 1 out]
                    n508 = Format Into String(format string="%.1f m/s" ("Format String"), w859) -> (resulting string=w861:string)  [unwired: 2 in, 1 out]
                    n509 = Build Array("LDA", w868, w861, w860) -> (w866:string[])
                    n510 = Build Array(w866, w865) -> (w864:string[][])
                  }
                }
              }
              frame #2 {
                n511 = global read "Meas_global.vi" "PWA Data"() -> (w881:T31)
                n512 = case shown="\"One Ch PWA\"" w881 {
                  tunnel: [string[][] [] w883] -> w880
                  frame "No PWA Data" {
                  }
                  frame "One Ch PWA" {
                    n513 = Build Array("PWA") -> (w884:string[])
                    n514 = Build Array(w884) -> (w883:string[][])
                  }
                }
              }
              frame #3 {
                n515 = global read "Meas_global.vi" "Acquisition vi to Run"() -> (w886:string)
                n516 = global read "Meas_global.vi" "Ch & spans"() -> (w888:T28[])
                n517 = for {
                  tunnel: w888 -> [w904] mode=indexing
                  tunnel: [w901] -> w887 mode=indexing
                  tunnel: w886 -> [w894]
                  n518 = Unbundle By Name(w904) -> ("DAQmx Chan"=w891:tag, "Var name"=w903:string, "Ch No"=w902:i16, "high limit (10V)"=w898:sgl, "low limit (-10V)"=w897:sgl)
                  n519 = Equal?(x=w894, y="NI-DAQmx.vi") -> (x = y?=w892:bool)
                  n520 = Number To Decimal String(number=w902) -> (decimal integer string=w890:string)  [unwired: 1 out]
                  n521 = Format Into String(format string="%.1f Volts" ("Format String"), w898) -> (resulting string=w896:string)  [unwired: 2 in, 1 out]
                  n522 = Format Into String(format string="%.1f Volts" ("Format String"), w897) -> (resulting string=w895:string)  [unwired: 2 in, 1 out]
                  n523 = Select(t=w891, s=w892, f=w890) -> (s? t:f=w889:string)
                  n524 = Build Array(w903, w889, w896, w895) -> (w901:string[])
                }
              }
              frame #4 {
                n525 = global read "Meas_global.vi" "Analysis Info cluster"() -> (w913:T22[])
                n526 = for {
                  tunnel: w913 -> [w923] mode=indexing
                  tunnel: [w922] -> w911 mode=indexing
                  n527 = Unbundle By Name(w923) -> ("Inst name"=w922:string)
                }
                n528 = global read "Meas_global.vi" "correlate"() -> (w912:i32[][])
                n529 = for {
                  tunnel: w912 -> [w918] mode=indexing
                  tunnel: w911 -> [w917]
                  tunnel: "Correlating" -> [w916]
                  tunnel: [w914] -> w906 mode=indexing
                  n530 = for {
                    tunnel: w918 -> [w921] mode=indexing
                    tunnel: w917 -> [w920]
                    tunnel: [w919] -> w915 mode=indexing
                    n531 = Index Array(array=w920, index=w921) -> (element=w919:string)
                  }
                  n532 = Build Array (concatenate)(w916, w915) -> (w914:string[])
                }
                n533 = Initialize Array("", 5 ("Dimension Size")) -> (w907:string[])
                n534 = Build Array (concatenate)(w907, w906) -> (w905:string[][])
              }
              frame #5 {
                n535 = Build Array (concatenate)(w929, w928, w924, w927, w925) -> (w926:string[][])
                n536 = local write "Statistics"(w926) -> ()
              }
              frame #6 {
                n537 = case shown="\"Take LDA data\"" w938 {
                  tunnel: [string[] [] w940] -> w935
                  frame "No LDA data" {
                  }
                  frame "Take LDA data" {
                    n538 = global read "Meas_global.vi" "Synchronise with LDA"() -> (w945:bool)
                    n539 = global read "Meas_global.vi" "Ch & spans"() -> (w948:T28[])
                    n540 = Array Size(array=w948) -> (size(s)=w947:i32)
                    n541 = Greater Than 0?(x=w947) -> (x > 0?=w946:bool)
                    n542 = Compound Arithmetic op=AND(w945, w946) -> (w944:bool)
                    n543 = Select(t="Synchronised with LDA", s=w944, f="") -> (s? t:f=w941:string)
                    n544 = Build Array(w941) -> (w940:string[])
                  }
                }
                n545 = global read "Meas_global.vi" "Continuous time trace?"() -> (w930:bool)
                n546 = Select(t="Continuous Time Trace", s=w930, f="") -> (s? t:f=w934:string)
                n547 = Build Array (concatenate)(w935, w934) -> (w933:string[])
                n548 = Build Array(w933) -> (w932:string[][])
                n549 = Transpose 2D Array(2D array=w932) -> (transposed array=w931:string[][])
                n550 = local write "Diagnostic info"(w931) -> ()
              }
            }
          }
        }
      }
      frame #18 {
        n551 = local read "File"() -> (w959:T5)
        n552 = Equal?(x=Setup."Run Program" ("setup"), y=w960) -> (x = y?=w957:bool)
        n553 = Not Equal?(x=w959, y=Save_Data."Save No Data" ("File")) -> (x != y?=w958:bool)
        n554 = global read "Meas_global.vi" "Repeat Measurement?"() -> (w949:bool)
        n555 = Compound Arithmetic op=AND(invert w949, w957, w958) -> (w956:bool)
        n556 = Get Date/Time In Seconds() -> (seconds since 1Jan1904=w953:timestamp)
        n557 = To Double Precision Float(number=w953) -> (double precision float=w951:dbl)
        n558 = local read "Setup filename"() -> (w954:string)
        n559 = case shown="True" w956 {
          tunnel: w959 -> [_ _]
          tunnel: w951 -> [w963 w996]
          tunnel: w954 -> [w962 w995]
          tunnel: w950 -> [w961 w994]
          frame True {
            n560 = stacked-sequence {
              seq-local: [_ w967 _] -> [_ _ w987]
              tunnel: w963 -> [w966 _ _]
              tunnel: w962 -> [w965 _ _]
              tunnel: w961 -> [w964 _ _]
              frame #0 {
                n561 = call "Write_Results_file.vi"("Experiment start time"=w964, "Experiment End time"=w966, "Setup filename"=w965) -> ()  [unwired: 4 out]
              }
              frame #1 {
                w972 = FALSE  # Empty list
                n562 = global read "Meas_global.vi" "Raw data file"() -> (w971:path)
                n563 = global read "Trav_pos_global.vi" "Top level setup filename"() -> (w969:path)
                n564 = global read "Meas_global.vi" "Start Time of experiment"() -> (w968:dbl)
                n565 = Strip Path(path=w971) -> (stripped path=w967:path)  [unwired: 1 out]
                n566 = Empty String/Path?(string/path=w969) -> (empty?=w970:bool)
                n567 = case shown="False" w970 {
                  tunnel: w969 -> [w986 _]
                  tunnel: w967 -> [w984 _]
                  tunnel: w968 -> [w982 _]
                  frame False {
                    n568 = call "Sec_to_date_filename.vi"("seconds"=w982) -> ("Day"=w981:string, "Time"=w980:string)  [unwired: 2 out]
                    n569 = Format Into String(format string="Cmd_%s_%s.xls", w981, w980) -> (resulting string=w978:string)  [unwired: 2 in, 1 out]
                    n570 = call "Fast_string_Replace.vi"("Replace match with:"="-", "Input String"=w978, "regular expression"=":") -> ("Output String"=w975:string)  [unwired: 2 out]
                    n571 = call "Fast_string_Replace.vi"("Replace match with:"="", "Input String"=w975, "regular expression"=" ") -> ("Output String"=w973:string)  [unwired: 2 out]
                    n572 = Build Path(base path=w984, name or relative path=w973) -> (appended path=w983:path)
                    n573 = Copy(10:w983, 11:w986) -> ()  [unwired: 1 in, 5 out]
                  }
                  frame True {
                  }
                }
                n574 = call "Remember_RD_Folders.vi"("Empty list"=w972, "Folders to Remember"=w967) -> ()  [unwired: 1 out]
              }
              frame #2 {
                n575 = global read "Meas_global.vi" "LDA data"() -> (w988:enum16{"No LDA data", "Take LDA data"})
                n576 = case shown="\"Take LDA data\"" w988 {
                  tunnel: w987 -> [_ w992]
                  frame "No LDA data" {
                  }
                  frame "Take LDA data" {
                    w990 = "LDA_Probe_Orientation.txt" ("name or relative path")
                    n577 = call "Setup_Filepath.vi"("Setup File Type"=Setup_Filetype."General", "Filename in"=w990) -> ("Filename Out"=w989:path)  [unwired: 1 out]
                    n578 = Build Path(base path=w992, name or relative path=w990) -> (appended path=w993:path)
                    n579 = Copy(10:w993, 11:w989) -> ()  [unwired: 1 in, 5 out]
                  }
                }
              }
            }
          }
          frame False {
            n580 = global read "Meas_global.vi" "Raw data option"() -> (w997:enum16{"Save raw data", "Raw data not saved"})
            n581 = case shown="\"Save raw data\"" w997 {
              tunnel: w994 -> [w1000 _]
              tunnel: w996 -> [w999 _]
              tunnel: w995 -> [w998 _]
              frame "Save raw data" {
                n582 = stacked-sequence {
                  tunnel: w1000 -> [_ w1009]
                  tunnel: w999 -> [_ w1008]
                  tunnel: w998 -> [_ w1006]
                  frame #0 {
                    n583 = global read "Meas_global.vi" "Current Block No"() -> (w1001:i32)
                    n584 = global write "Meas_global.vi" "Requested No of blocks"(w1001) -> ()
                  }
                  frame #1 {
                    n585 = call "Create_Raw_data_file.vi"("No of averages"=1, "End time"=w1008, "Start time"=w1009, "Setup filename"=w1006) -> ("Values"=w1004:string[][], "Column headers"=w1005:string[])  [unwired: 2 out]
                    n586 = Index Array(array=w1004, index (row)=0) -> (element=w1002:string[])  [unwired: 1 in]
                    n587 = global write "Dynamic_call_global.ph.vi" "Plug in values"(w1002) -> ()
                    n588 = global write "Dynamic_call_global.ph.vi" "Plug in titles"(w1005) -> ()
                  }
                }
              }
              frame "Raw data not saved" {
              }
            }
          }
        }
      }
      frame #19 {
        n589 = stacked-sequence {
          seq-local: [w1016 _] -> [_ w1025]
          seq-local: [w1012 _] -> [_ w1024]
          tunnel: w1010 -> [w1023 _]
          frame #0 {
            n590 = global read "Meas_global.vi" "Raw data file"() -> (w1014:path)
            n591 = global read "Meas_global.vi" "Raw data option"() -> (w1022:enum16{"Save raw data", "Raw data not saved"})
            n592 = Equal?(x=Setup."Run Program" ("setup"), y=w1023) -> (x = y?=w1018:bool)
            n593 = Strip Path(path=w1014) -> (stripped path=w1013:path)  [unwired: 1 out]
            n594 = Equal?(x=w1022, y=enum16{"Save raw data", "Raw data not saved"}."Save raw data" ("Raw data option")) -> (x = y?=w1017:bool)
            n595 = Build Path(base path=w1013, name or relative path="VI_History.xls") -> (appended path=w1012:path)
            n596 = call "Does_file_exist_(simple).vi"("Pathname"=w1012) -> ("exists?"=w1020:bool)
            n597 = Not(x=w1020) -> (.not. x?=w1019:bool)
            n598 = Compound Arithmetic op=AND(w1019, w1018, w1017) -> (w1016:bool)
          }
          frame #1 {
            n599 = case shown="True" w1025 {
              tunnel: w1024 -> [_ w1026]
              frame False {
              }
              frame True {
                n600 = stacked-sequence {
                  tunnel: w1026 -> [w1032 w1040]
                  frame #0 {
                    w1029 = FALSE  # Lock File
                    n601 = global read "Meas_global.vi" "ProgRevisionInfo"() -> (w1028:string)
                    n602 = call "Characters_to_string.vi"("Characters to write"=w1028, "Label for characters"="Prog Revision info") -> ("Output string"=w1034:string)
                    n603 = call "Date_and_Time_to_string.vi"() -> ("Date and time (spreadsheet)"=w1035:string)
                    n604 = call "Get_mod_dates.vi"() -> ("error out"=w1033:errorcluster, "Output string"=w1030:string)  [unwired: 1 in, 3 out]
                    n605 = call "EnFlo_Error_Handler.vi"("error in (no error)"=w1033) -> ()  [unwired: 2 in, 3 out]
                    n606 = Concatenate Strings(w1035, w1034, w1030) -> (w1031:string)
                    n607 = call "Write_Characters_To_File.vi"("file path (dialog if empty)"=w1032, "character string"=w1031, "Lock File"=w1029) -> ()  [unwired: 2 in, 4 out]
                  }
                  frame #1 {
                    n608 = global read "Trav_pos_global.vi" "Traverses to Move"() -> (w1038:string[])
                    n609 = global read "Constants_global.vi" "Traverse folder"() -> (w1039:path)
                    n610 = Strip Path(path=w1040) -> (stripped path=w1037:path)  [unwired: 1 out]
                    n611 = for {
                      tunnel: w1039 -> [w1052]
                      tunnel: w1038 -> [w1048] mode=indexing
                      tunnel: w1037 -> [w1049]
                      tunnel: string[] ["Traverse_Preferences.txt", "Traverse_Setup.xls"] ("Traverses to Move") -> [w1041]
                      n612 = Build Path(base path=w1052, name or relative path=w1048) -> (appended path=w1044:path)
                      n613 = Build Path(base path=w1044, name or relative path="Trav_Space_Files" ("Substring")) -> (appended path=w1051:path)
                      n614 = Build Path(base path=w1051, name or relative path="Selected_Filename.txt" ("Substring")) -> (appended path=w1056:path)
                      n615 = call "Create_directory_path.vi"("Path name"=w1056) -> ("Path name Out"=w1055:path)  [unwired: 1 in, 1 out]
                      n616 = Build Path(base path=w1049, name or relative path=w1048) -> (appended path=w1043:path)
                      n617 = for {
                        tunnel: w1044 -> [w1063]
                        tunnel: w1043 -> [w1061]
                        tunnel: w1041 -> [w1059] mode=indexing
                        n618 = Build Path(base path=w1063, name or relative path=w1059) -> (appended path=w1062:path)
                        n619 = Build Path(base path=w1061, name or relative path=w1059) -> (appended path=w1058:path)
                        n620 = call "Create_directory_path.vi"("Path name"=w1058) -> ("Path name Out"=w1057:path)  [unwired: 1 in, 1 out]
                        n621 = Copy(9:TRUE ("overwrite (F)"), 10:w1057, 11:w1062) -> ()  [unwired: 2 in, 3 out]
                      }
                      n622 = call "Read_File_Simple.vi"("Filename"=w1055) -> ("string"=w1046:string)  [unwired: 2 in, 7 out]
                      n623 = Build Path(base path=w1043, name or relative path=w1046) -> (appended path=w1047:path)
                      n624 = Build Path(base path=w1051, name or relative path=w1046) -> (appended path=w1050:path)
                      n625 = call "Create_directory_path.vi"("Path name"=w1047) -> ("Path name Out"=w1045:path)  [unwired: 1 in, 1 out]
                      n626 = Copy(9:TRUE ("overwrite (F)"), 10:w1045, 11:w1050) -> ()  [unwired: 2 in, 3 out]
                    }
                  }
                }
              }
            }
          }
        }
      }
      frame #20 {
        n627 = local read "Correlate?"() -> (w1068:T9)
        n628 = case shown="\"Run Program\"" w1065 {
          tunnel: w1065 -> [w1070 _ _ _]
          tunnel: [w1070 w1083 w1084 w1085] -> w1064
          frame "Run Program" {
            n629 = global read "Meas_global.vi" "Analysis Info cluster"() -> (w1069:T22[])
            n630 = for {
              tunnel: w1069 -> [w1081] mode=indexing
              stop <- w1071 stop-if-true
              w1078 = "Pitot ("
              n631 = Unbundle By Name(w1081) -> ("U"=w1072:dbl, "Inst name"=w1077:string)
              n632 = String Length(string=w1078) -> (length=w1080:i32)
              n633 = String Subset(string=w1077, length (rest)=w1080) -> (substring=w1079:string)  [unwired: 1 out]
              n634 = Equal?(x=w1079, y=w1078) -> (x = y?=w1074:bool)
              n635 = call "Match_Pat_Case_In.vi"("String to match"="ref", "String"=w1077) -> ("offset past match"=w1075:i32)  [unwired: 1 in, 3 out]
              n636 = Greater Or Equal To 0?(x=w1075) -> (x >= 0?=w1073:bool)
              n637 = And(x=w1073, y=w1074) -> (x .and. y?=w1071:bool)
              n638 = case shown="True" w1071 {
                tunnel: w1072 -> [_ w1082]
                frame False {
                }
                frame True {
                  n639 = call "Log_Reference_Velocity.vi"("Measured Velocity"=w1082) -> ()  [unwired: 1 out]
                }
              }
            }
          }
          frame "Show Setup" {
            w1083 = Setup."Run Program"  # setup
          }
          frame "Save Current Setup" {
            w1084 = Setup."Run Program"  # setup
          }
          frame "Setup Front Panel" {
            w1085 = Setup."Run Program"  # setup
          }
        }
        n640 = case shown="\"Correlate without activating panel\"" w1068 {
          tunnel: [T9."Cross correlation off" T9."Correlate without activating panel" T9."Correlate without activating panel"] -> w1067
          frame "Cross correlation off" {
          }
          frame "Show correlation panel" {
          }
          frame "Correlate without activating panel" {
          }
        }
        n641 = local write "Correlate?"(w1067) -> ()
        n642 = global write "Meas_global.vi" "Remote control"(FALSE ("Remote control")) -> ()
        n643 = call "Program_Active.vi"() -> ()  [unwired: 1 in]
        n644 = local write "setup"(w1064) -> ()
      }
      frame #21 {
        w1094 = FALSE  # Dialog Box (T)
        n645 = global read "Meas_global.vi" "Post Process"() -> (w1089:T2)
        n646 = case shown="\"Take New Data\"" w1089 {
          frame "Take New Data" {
            n647 = global read "Meas_global.vi" "Analysis Info cluster"() -> (w1106:T22[])
            n648 = global read "Meas_global.vi" "Requested Sampling rate"() -> (w1105:dbl)
            n649 = Divide(x=w1105, y=10.0) -> (x/y=w1098:dbl)
            n650 = Max & Min(x=w1098, y=100.0) -> (min(x,y)=w1097:dbl)  [unwired: 1 out]
            n651 = for {
              tunnel: w1106 -> [w1133] mode=indexing
              tunnel: w1097 -> [w1127]
              tunnel: [w1129] -> w1103
              tunnel: [w1128] -> w1101
              tunnel: [w1126] -> w1100
              stop <- w1129 stop-if-true
              n652 = Unbundle By Name(w1133) -> ("Inst name"=w1128:string, "Av Sampling Rate"=w1126:dbl, "Inst type"=w1132:T16)
              n653 = Equal?(x=w1132, y=Inst_type."LDA Vel" ("Inst type")) -> (x = y?=w1130:bool)
              n654 = Less?(x=w1126, y=w1127) -> (x < y?=w1125:bool)
              n655 = Greater Than 0?(x=w1126) -> (x > 0?=w1124:bool)
              n656 = Compound Arithmetic op=AND(w1125, w1124, w1130) -> (w1129:bool)
            }
            n657 = case shown="True" w1103 {
              tunnel: [FALSE w1108] -> w1102
              frame False {
              }
              frame True {
                n658 = global read "Preference_global.vi" "Rig Setup"() -> (w1114:string)
                n659 = Concatenate Strings("Status:of:", w1114) -> (w1113:string)
                n660 = Build Array(w1113) -> (w1112:string[])
                n661 = call "Get_Current_Scan_client.vi"("ADAM Ch Names"=w1112) -> ("Numerical Values"=w1111:dbl[])  [unwired: 1 in, 2 out]
                n662 = Index Array(array=w1111) -> (element=w1110:dbl)  [unwired: 1 in]
                n663 = Equal?(x=2.0, y=w1110) -> (x = y?=w1108:bool)
              }
            }
            n664 = case shown="True" w1102 {
              tunnel: w1101 -> [_ w1119]
              tunnel: w1100 -> [_ w1117]
              frame False {
              }
              frame True {
                w1122 = FALSE  # Dialog Box (T)
                n665 = Format Into String(format string="The %s currently has a data rate of %d Hz", w1119, w1117) -> (resulting string=w1118:string)  [unwired: 2 in, 1 out]
                n666 = Bundle By Name(cluster=errorcluster {"status"=TRUE, "code"=0, "source"=""} ("error in (no error)"), "source"=w1118) -> (w1121:errorcluster)
                n667 = call "EnFlo_Error_Handler.vi"("error in (no error)"=w1121, "Error Type"="Low LDA Sampling Rate", "Dialog Box (T)"=w1122) -> ()  [unwired: 3 out]
              }
            }
          }
          frame "Post Process Raw Data File" {
          }
        }
        n668 = global read "Meas_global.vi" "Over/Under string"() -> (w1092:string)
        n669 = Empty String/Path?(string/path=w1092) -> (empty?=w1091:bool)
        n670 = Not(x=w1091) -> (.not. x?=w1090:bool)
        n671 = Bundle By Name(cluster=errorcluster {"status"=FALSE, "code"=0, "source"=""} ("error in (no error)"), "source"=w1092, "status"=w1090) -> (w1095:errorcluster)
        n672 = call "EnFlo_Error_Handler.vi"("error in (no error)"=w1095, "Error Type"="Signal Clipping", "Dialog Box (T)"=w1094) -> ()  [unwired: 3 out]
      }
      frame #22 {
        w1136 = string[] [] ("Per Block Plug Ins Extra")
        n673 = Empty String/Path?(string/path=w1140) -> (empty?=w1139:bool)
        n674 = global read "Dynamic_call_global.ph.vi" "Final Plug Ins"() -> (w1141:string[])
        n675 = case shown="True" w1139 {
          tunnel: w1140 -> [w1152 _]
          frame False {
            n676 = local read "Comments"() -> (w1151:string)
            n677 = call "Fast_string_Replace.vi"("Replace match with:"="", "Input String"=w1151, "regular expression"=w1152) -> ("Output String"=w1150:string)  [unwired: 2 out]
            n678 = local write "Comments"(w1150) -> ()
          }
          frame True {
          }
        }
        n679 = call "Plug_in_Directories.vi"() -> ("Final"=w1137:path)  [unwired: 3 out]
        n680 = for {
          tunnel: w1141 -> [w1155] mode=indexing
          tunnel: w1137 -> [w1154]
          w1158 = FALSE  # Dialog Box (T)
          n681 = Build Path(base path=w1154, name or relative path=w1155) -> (appended path=w1153:path)
          n682 = global read "Dynamic_call_global.ph.vi" "Plug in"() -> (w1163:refnum<vi>)
          n683 = Open VI Reference(type specifier VI Refnum (for type only)=w1163, vi path=w1153) -> (vi reference=w1162:refnum<vi>, error out=w1161:errorcluster)  [unwired: 2 in, 2 out]
          n684 = call-by-ref "?"(reference=w1162, error in=w1161) -> (reference out=w1159:refnum<vi>, error out=w1160:errorcluster)  [unwired: 6 in, 2 out]
          n685 = Close Reference(reference=w1159, error in (no error)=w1160) -> (error out=w1156:errorcluster)
          n686 = call "EnFlo_Error_Handler.vi"("error in (no error)"=w1156, "Error Type"="Running Final Plug In", "Dialog Box (T)"=w1158) -> ()  [unwired: 3 out]
        }
        n687 = global read "Meas_global.vi" "Repeat Measurement?"() -> (w1138:bool)
        n688 = case shown="True" w1138 {
          tunnel: w1135 -> [_ w1148]
          tunnel: [FALSE w1143] -> w1134
          frame False {
          }
          frame True {
            n689 = global read "Meas_global.vi" "Post Process"() -> (w1146:T2)
            n690 = Equal To 0?(x=w1148) -> (x = 0?=w1144:bool)
            n691 = Equal?(x=w1146, y=Post_Process."Post Process Raw Data File" ("Post Process")) -> (x = y?=w1145:bool)
            n692 = And(x=w1145, y=w1144) -> (x .and. y?=w1143:bool)
          }
        }
        n693 = global write "Dynamic_call_global.ph.vi" "Per Block Plug Ins Extra"(w1136) -> ()
        n694 = global write "Dynamic_call_global.ph.vi" "Initial Plug Ins Extra"(w1136) -> ()
      }
      frame #23 {
        n695 = global read "Meas_global.vi" "Post Process"() -> (w1170:T2)
        n696 = local read "stop"() -> (w1176:bool)
        n697 = Equal?(x=w1171, y=Setup."Run Program" ("setup")) -> (x = y?=w1167:bool)
        n698 = Equal?(x=w1170, y=Post_Process."Take New Data" ("Post Process")) -> (x = y?=w1168:bool)
        n699 = And(x=w1167, y=w1168) -> (x .and. y?=w1166:bool)
        n700 = case shown="False" w1176 {
          tunnel: [Multi_Run_Status."Continue" ("Status Out") Multi_Run_Status."Terminate Run" ("Status Out")] -> w1174
          frame False {
          }
          frame True {
            n701 = local write "stop"(FALSE) -> ()
          }
        }
        n702 = case shown="True" w1166 {
          tunnel: w1174 -> [w1177 w1181]
          tunnel: [w1177 w1183] -> w1173
          frame False {
          }
          frame True {
            n703 = local read "Raw data file"() -> (w1182:path)
            n704 = global read "Meas_global.vi" "Acquisition vi Ref"() -> (w1178:refnum<vi>)
            n705 = Path to Array of Strings(0:w1182) -> (2:w1184:string[])  [unwired: 1 out]
            n706 = Index Array(array=w1184, index=0 ("Index")) -> (element=w1180:string)
            n707 = Close Reference(reference=w1178) -> ()  [unwired: 1 in, 1 out]
            n708 = Build Array(w1180) -> (w1179:string[])
            n709 = for {
              tunnel: w1179 -> [w1188] mode=indexing
              shift-right: [w1186] -> w1183
              shift-left: w1181 -> [w1187]
              n710 = call "Warn_on_low_HD_space.vi"("Status In"=w1187, "HD name"=w1188) -> ("Status Out"=w1186:T1)  [unwired: 6 out]
            }
          }
        }
        "Status Out" <- w1173
        n711 = global write "Trav_pos_global.vi" "Dummy Measurement?"(FALSE ("Dummy Measurement?")) -> ()
        n712 = global write "Plug_in_data_global.vi" "Server Channels to log"(string[] [] ("Server Channels to log")) -> ()
        n713 = global write "Meas_global.vi" "Extra Comments"("") -> ()
      }
    }
  }
